vi "C-V measurement.vi"(5 "Session properties":T2, 7 "Workspace":path, 8 "Error In":errorcluster, 9 "myDLTS file path":path=path "", 10 "CV measurement":T22 {"CV properties"."Equivalent circuit model" items=["Rp || Cp", "Rs + Cs", "Rs + Ls", "G B", "D Cs", "Q Cs", "D Ls", "Q Ls", "Rp || Lp", "D Cp"]; "CV properties"."V range" items=["10mV"=0.01, "100mV"=0.1, "1V"=1.0, "10V"=10.0]; "CV properties"."I range" items=["100nA"=-7.0, "1µA"=-6.0, "10µA"=-5.0, "100µA"=-4.0, "1mA"=-3.0, "10mA"=-2.0]}, 11 "Loop data":T3={"Persistent"={"Last file"=path "", "Last user"="", "Users"=[]}, "Temp handle"={"Connected"=FALSE, "Temp ctrl"={"Gain (P)"=0.0, "Reset (I)"=0.0, "Rate (D)"=0.0, "Stabilization rate"=0.0, "Stabilization delta"=0.0, "Type"=enum."Lake Shore 325", "Custom temp ctrl"={"VISA resource name"=""}, "Lakeshore 325"={"VISA name"="", "Loop"=0, "Heater Range"=1, "Heater Resistance"=0, "Sample sensor"=0, "Fast sensor"=0, "Slow sensor"=0}, "Lakeshore 331"={"VISA name"="", "Loop"=1, "Heater Range"=0, "Sample sensor"=0, "Fast sensor"=0, "Slow sensor"=0}, "Lakeshore 332"={"VISA name"="", "Loop"=1, "Heater Range"=0, "Sample sensor"=0, "Fast sensor"=0, "Slow sensor"=0}, "Lakeshore 335"={"VISA name"="", "Loop"=1, "Sample sensor"=0, "Fast sensor"=0, "Slow sensor"=0, "Heater Range"=0, "Output mode"=enum."Off"}, "Lakeshore 336"={"VISA name"="", "Loop"=1, "Output mode"=enum."Off", "Max current"=1.0, "Heater resistance"=1, "Sample sensor"=1, "Slow sensor"=1, "Fast sensor"=1}}}, "Paths"={"Manual"=path "", "Settings"=path "", "Persistent"=path "", "Work dir."=path ""}, "Settings"={"MFIA"={"Address"="", "Use compensation"=TRUE, "Shut down gracefully"=FALSE}, "Temp ctrl"={"Gain (P)"=0.0, "Reset (I)"=0.0, "Rate (D)"=0.0, "Stabilization rate"=0.0, "Stabilization delta"=0.0, "Type"=enum."Lake Shore 325", "Custom temp ctrl"={"VISA resource name"=""}, "Lakeshore 325"={"VISA name"="", "Loop"=0, "Heater Range"=1, "Heater Resistance"=0, "Sample sensor"=0, "Fast sensor"=0, "Slow sensor"=0}, "Lakeshore 331"={"VISA name"="", "Loop"=1, "Heater Range"=0, "Sample sensor"=0, "Fast sensor"=0, "Slow sensor"=0}, "Lakeshore 332"={"VISA name"="", "Loop"=1, "Heater Range"=0, "Sample sensor"=0, "Fast sensor"=0, "Slow sensor"=0}, "Lakeshore 335"={"VISA name"="", "Loop"=1, "Sample sensor"=0, "Fast sensor"=0, "Slow sensor"=0, "Heater Range"=0, "Output mode"=enum."Off"}, "Lakeshore 336"={"VISA name"="", "Loop"=1, "Output mode"=enum."Off", "Max current"=1.0, "Heater resistance"=1, "Sample sensor"=1, "Slow sensor"=1, "Fast sensor"=1}}, "Source-meter"={"Type"=enum."Custom", "Custom source-meter"={"VISA resource name"=""}, "Keithley 2600"={"VISA name"="", "Ignore ID Query"=FALSE, "SMU"=enum."Channel A"}, "Keithley 2400 Series"={"VISA name"="", "Ignore ID Query"=FALSE}}, "Other"={"Enable OriginLab"=FALSE, "Reader mode"=FALSE, "Auto-save"=FALSE}, "Defaults"={"IV properties"={"T"=0.0, "Vstart"=-0.5, "Vstop"=0.5, "Vpoints"=10.0, "Settling"=0.01, "I limit"=0.1, "Log mapping"=FALSE, "Averaging"=0.0}, "CV properties"={"T"=0.0, "Vstart"=-0.5, "Vstop"=0.5, "Vpoints"=10.0, "Precision"=enum."Normal", "Test signal"=0.01, "Auto I range"=FALSE, "Test frequency"=100000.0, "I range"=-2.0, "V range"=10.0, "Log mapping"=FALSE, "Rel perm"=0.0, "Area"=0.0, "Equivalent circuit model"=0}, "DLTS properties"={"Tstart"=0.0, "Instant start"=FALSE, "Tstop"=0.0, "T rate"=0.0, "Test signal"=0.0, "Test frequency"=0.0, "Bandwidth"=0.0, "Averaging"=0.0, "Vbias"=0.0, "Vpulse"=0.0, "pulse length"=0.0, "Pulse 2"=FALSE, "Vpulse 2"=0.0, "pulse length 2"=0.0, "I range"=-2.0, "V range"=10.0, "Emission rate"=[], "Sampling rate"=0.0, "Acq. delay"=0.0, "Filter order"=0, "Equivalent circuit model"=0}, "LDLTS properties"={"T"=0.0, "Test signal"=0.0, "Test frequency"=0.0, "Bandwidth"=0.0, "Averaging"=0.0, "Vbias"=0.0, "Vpulse"=0.0, "pulse length"=0.0, "Pulse 2"=FALSE, "Vpulse 2"=0.0, "pulse length 2"=0.0, "I range"=-2.0, "V range"=10.0, "Sampling rate"=0.0, "Acq. delay"=0.0, "Sampling time"=0.0, "Filter order"=0, "Equivalent circuit model"=0}}}, "Software version"=0.0, "MFIA handle"={"ziHandle"={"handleValid"=FALSE, "Conn"=0, "Path Prefix"="", "Handle"=0, "Connected"=FALSE, "Clockbase(s)"=0.0}, "Selected device"="", "ziModHandle"={"handleValid"=FALSE, "Conn"=0, "ModHandle"=0, "moduleID"="", "Path Prefix"=""}}, "Source-meter handle"={"Connected"=FALSE, "Source-meter"={"Type"=enum."Custom", "Custom source-meter"={"VISA resource name"=""}, "Keithley 2600"={"VISA name"="", "Ignore ID Query"=FALSE, "SMU"=enum."Channel A"}, "Keithley 2400 Series"={"VISA name"="", "Ignore ID Query"=FALSE}}}} {"MFIA handle"."ziModHandle"."ModHandle" format="0x%08x"; "MFIA handle"."ziModHandle"."Conn" format="0x%08x"; "MFIA handle"."ziHandle"."Handle" format="0x%08x"; "MFIA handle"."ziHandle"."Conn" format="0x%08x"; "Settings"."Defaults"."LDLTS properties"."Equivalent circuit model" items=["Rp || Cp", "Rs + Cs", "Rs + Ls", "G B", "D Cs", "Q Cs", "D Ls", "Q Ls", "Rp || Lp", "D Cp"]; "Settings"."Defaults"."LDLTS properties"."Filter order" min=0 max=8 step=1; "Settings"."Defaults"."LDLTS properties"."Sampling rate" items=["13k"=13392.857422, "27k"=26785.714844, "54k"=53571.429687, "107k"=107142.859375]; "Settings"."Defaults"."LDLTS properties"."V range" items=["10mV"=0.01, "100mV"=0.1, "1V"=1.0, "10V"=10.0]; "Settings"."Defaults"."LDLTS properties"."I range" items=["100nA"=-7.0, "1µA"=-6.0, "10µA"=-5.0, "100µA"=-4.0, "1mA"=-3.0, "10mA"=-2.0]; "Settings"."Defaults"."DLTS properties"."Equivalent circuit model" items=["Rp || Cp", "Rs + Cs", "Rs + Ls", "G B", "D Cs", "Q Cs", "D Ls", "Q Ls", "Rp || Lp", "D Cp"]; "Settings"."Defaults"."DLTS properties"."Filter order" min=0 max=8 step=1; "Settings"."Defaults"."DLTS properties"."Sampling rate" items=["13k"=13392.857422, "27k"=26785.714844, "54k"=53571.429687, "107k"=107142.859375]; "Settings"."Defaults"."DLTS properties"."V range" items=["10mV"=0.01, "100mV"=0.1, "1V"=1.0, "10V"=10.0]; "Settings"."Defaults"."DLTS properties"."I range" items=["10mV"=0.01, "100mV"=0.1, "1V"=1.0, "10V"=10.0]; "Settings"."Defaults"."CV properties"."Equivalent circuit model" items=["Rp || Cp", "Rs + Cs", "Rs + Ls", "G B", "D Cs", "Q Cs", "D Ls", "Q Ls", "Rp || Lp", "D Cp"]; "Settings"."Defaults"."CV properties"."V range" items=["10mV"=0.01, "100mV"=0.1, "1V"=1.0, "10V"=10.0]; "Settings"."Defaults"."CV properties"."I range" items=["100nA"=-7.0, "1µA"=-6.0, "10µA"=-5.0, "100µA"=-4.0, "1mA"=-3.0, "10mA"=-2.0]; "Settings"."Defaults"."IV properties"."Settling" min=0.0 max=65535.0; "Settings"."Temp ctrl"."Lakeshore 336"."Fast sensor" items=["Sensor A", "Sensor B", "Sensor C", "Sensor D"]; "Settings"."Temp ctrl"."Lakeshore 336"."Slow sensor" items=["Sensor A", "Sensor B", "Sensor C", "Sensor D"]; "Settings"."Temp ctrl"."Lakeshore 336"."Sample sensor" items=["Sensor A", "Sensor B", "Sensor C", "Sensor D"]; "Settings"."Temp ctrl"."Lakeshore 336"."Heater resistance" items=["25 Ohm"=1, "50 Ohm"=2]; "Settings"."Temp ctrl"."Lakeshore 336"."Max current" items=["0.707 A"=0.0, "1 A"=1.0, "1.414 A"=1.414, "2 A"=2.0]; "Settings"."Temp ctrl"."Lakeshore 336"."Loop" items=["Output 1"=1, "Output 2"=2, "Output 3"=3, "Output 4"=4]; "Settings"."Temp ctrl"."Lakeshore 335"."Heater Range" items=["Off", "Low (On)", "Medium", "High"]; "Settings"."Temp ctrl"."Lakeshore 335"."Slow sensor" items=["A", "B"]; "Settings"."Temp ctrl"."Lakeshore 335"."Fast sensor" items=["A", "B"]; "Settings"."Temp ctrl"."Lakeshore 335"."Sample sensor" items=["A", "B"]; "Settings"."Temp ctrl"."Lakeshore 335"."Loop" items=["Loop 1"=1, "Loop 2"=2]; "Settings"."Temp ctrl"."Lakeshore 332"."Slow sensor" items=["A", "B"]; "Settings"."Temp ctrl"."Lakeshore 332"."Fast sensor" items=["A", "B"]; "Settings"."Temp ctrl"."Lakeshore 332"."Sample sensor" items=["A", "B"]; "Settings"."Temp ctrl"."Lakeshore 332"."Heater Range" items=["Off", "Low (0.5W)", "Med (5W)", "High (50W)"]; "Settings"."Temp ctrl"."Lakeshore 332"."Loop" items=["Loop 1", "Loop 2"]; "Settings"."Temp ctrl"."Lakeshore 331"."Slow sensor" items=["A", "B"]; "Settings"."Temp ctrl"."Lakeshore 331"."Fast sensor" items=["A", "B"]; "Settings"."Temp ctrl"."Lakeshore 331"."Sample sensor" items=["A", "B"]; "Settings"."Temp ctrl"."Lakeshore 331"."Heater Range" items=["Off", "Low (0.5W)", "Med (5W)", "High (50W)"]; "Settings"."Temp ctrl"."Lakeshore 331"."Loop" items=["Loop 1", "Loop 2"]; "Settings"."Temp ctrl"."Lakeshore 325"."Slow sensor" items=["A", "B"]; "Settings"."Temp ctrl"."Lakeshore 325"."Fast sensor" items=["A", "B"]; "Settings"."Temp ctrl"."Lakeshore 325"."Sample sensor" items=["A", "B"]; "Settings"."Temp ctrl"."Lakeshore 325"."Heater Resistance" items=["25 Ohm"=1, "50 Ohm"=2]; "Settings"."Temp ctrl"."Lakeshore 325"."Heater Range" items=["Off", "Low (loop 1) or On (loop 2)", "High (loop 1)"]; "Settings"."Temp ctrl"."Lakeshore 325"."Loop" items=["Loop 1"=1, "Loop 2"=2]; "Temp handle"."Temp ctrl"."Lakeshore 336"."Fast sensor" items=["Sensor A", "Sensor B", "Sensor C", "Sensor D"]; "Temp handle"."Temp ctrl"."Lakeshore 336"."Slow sensor" items=["Sensor A", "Sensor B", "Sensor C", "Sensor D"]; "Temp handle"."Temp ctrl"."Lakeshore 336"."Sample sensor" items=["Sensor A", "Sensor B", "Sensor C", "Sensor D"]; "Temp handle"."Temp ctrl"."Lakeshore 336"."Heater resistance" items=["25 Ohm"=1, "50 Ohm"=2]; "Temp handle"."Temp ctrl"."Lakeshore 336"."Max current" items=["0.707 A"=0.0, "1 A"=1.0, "1.414 A"=1.414, "2 A"=2.0]; "Temp handle"."Temp ctrl"."Lakeshore 336"."Loop" items=["Output 1"=1, "Output 2"=2, "Output 3"=3, "Output 4"=4]; "Temp handle"."Temp ctrl"."Lakeshore 335"."Heater Range" items=["Off", "Low (On)", "Medium", "High"]; "Temp handle"."Temp ctrl"."Lakeshore 335"."Slow sensor" items=["A", "B"]; "Temp handle"."Temp ctrl"."Lakeshore 335"."Fast sensor" items=["A", "B"]; "Temp handle"."Temp ctrl"."Lakeshore 335"."Sample sensor" items=["A", "B"]; "Temp handle"."Temp ctrl"."Lakeshore 335"."Loop" items=["Loop 1"=1, "Loop 2"=2]; "Temp handle"."Temp ctrl"."Lakeshore 332"."Slow sensor" items=["A", "B"]; "Temp handle"."Temp ctrl"."Lakeshore 332"."Fast sensor" items=["A", "B"]; "Temp handle"."Temp ctrl"."Lakeshore 332"."Sample sensor" items=["A", "B"]; "Temp handle"."Temp ctrl"."Lakeshore 332"."Heater Range" items=["Off", "Low (0.5W)", "Med (5W)", "High (50W)"]; "Temp handle"."Temp ctrl"."Lakeshore 332"."Loop" items=["Loop 1", "Loop 2"]; "Temp handle"."Temp ctrl"."Lakeshore 331"."Slow sensor" items=["A", "B"]; "Temp handle"."Temp ctrl"."Lakeshore 331"."Fast sensor" items=["A", "B"]; "Temp handle"."Temp ctrl"."Lakeshore 331"."Sample sensor" items=["A", "B"]; "Temp handle"."Temp ctrl"."Lakeshore 331"."Heater Range" items=["Off", "Low (0.5W)", "Med (5W)", "High (50W)"]; "Temp handle"."Temp ctrl"."Lakeshore 331"."Loop" items=["Loop 1", "Loop 2"]; "Temp handle"."Temp ctrl"."Lakeshore 325"."Slow sensor" items=["A", "B"]; "Temp handle"."Temp ctrl"."Lakeshore 325"."Fast sensor" items=["A", "B"]; "Temp handle"."Temp ctrl"."Lakeshore 325"."Sample sensor" items=["A", "B"]; "Temp handle"."Temp ctrl"."Lakeshore 325"."Heater Resistance" items=["25 Ohm"=1, "50 Ohm"=2]; "Temp handle"."Temp ctrl"."Lakeshore 325"."Heater Range" items=["Off", "Low (loop 1) or On (loop 2)", "High (loop 1)"]; "Temp handle"."Temp ctrl"."Lakeshore 325"."Loop" items=["Loop 1"=1, "Loop 2"=2]}) -> (0 "Error Out":errorcluster, 1 "Modified":bool, 2 "CV measurement out":T22 {"CV properties"."Equivalent circuit model" items=["Rp || Cp", "Rs + Cs", "Rs + Ls", "G B", "D Cs", "Q Cs", "D Ls", "Q Ls", "Rp || Lp", "D Cp"]; "CV properties"."V range" items=["10mV"=0.01, "100mV"=0.1, "1V"=1.0, "10V"=10.0]; "CV properties"."I range" items=["100nA"=-7.0, "1µA"=-6.0, "10µA"=-5.0, "100µA"=-4.0, "1mA"=-3.0, "10mA"=-2.0]}, 3 "Loop data out":T3={"Persistent"={"Last file"=path "", "Last user"="", "Users"=[]}, "Temp handle"={"Connected"=FALSE, "Temp ctrl"={"Gain (P)"=0.0, "Reset (I)"=0.0, "Rate (D)"=0.0, "Stabilization rate"=0.0, "Stabilization delta"=0.0, "Type"=enum."Lake Shore 325", "Custom temp ctrl"={"VISA resource name"=""}, "Lakeshore 325"={"VISA name"="", "Loop"=0, "Heater Range"=1, "Heater Resistance"=0, "Sample sensor"=0, "Fast sensor"=0, "Slow sensor"=0}, "Lakeshore 331"={"VISA name"="", "Loop"=1, "Heater Range"=0, "Sample sensor"=0, "Fast sensor"=0, "Slow sensor"=0}, "Lakeshore 332"={"VISA name"="", "Loop"=1, "Heater Range"=0, "Sample sensor"=0, "Fast sensor"=0, "Slow sensor"=0}, "Lakeshore 335"={"VISA name"="", "Loop"=1, "Sample sensor"=0, "Fast sensor"=0, "Slow sensor"=0, "Heater Range"=0, "Output mode"=enum."Off"}, "Lakeshore 336"={"VISA name"="", "Loop"=1, "Output mode"=enum."Off", "Max current"=1.0, "Heater resistance"=1, "Sample sensor"=1, "Slow sensor"=1, "Fast sensor"=1}}}, "Paths"={"Manual"=path "", "Settings"=path "", "Persistent"=path "", "Work dir."=path ""}, "Settings"={"MFIA"={"Address"="", "Use compensation"=TRUE, "Shut down gracefully"=FALSE}, "Temp ctrl"={"Gain (P)"=0.0, "Reset (I)"=0.0, "Rate (D)"=0.0, "Stabilization rate"=0.0, "Stabilization delta"=0.0, "Type"=enum."Lake Shore 325", "Custom temp ctrl"={"VISA resource name"=""}, "Lakeshore 325"={"VISA name"="", "Loop"=0, "Heater Range"=1, "Heater Resistance"=0, "Sample sensor"=0, "Fast sensor"=0, "Slow sensor"=0}, "Lakeshore 331"={"VISA name"="", "Loop"=1, "Heater Range"=0, "Sample sensor"=0, "Fast sensor"=0, "Slow sensor"=0}, "Lakeshore 332"={"VISA name"="", "Loop"=1, "Heater Range"=0, "Sample sensor"=0, "Fast sensor"=0, "Slow sensor"=0}, "Lakeshore 335"={"VISA name"="", "Loop"=1, "Sample sensor"=0, "Fast sensor"=0, "Slow sensor"=0, "Heater Range"=0, "Output mode"=enum."Off"}, "Lakeshore 336"={"VISA name"="", "Loop"=1, "Output mode"=enum."Off", "Max current"=1.0, "Heater resistance"=1, "Sample sensor"=1, "Slow sensor"=1, "Fast sensor"=1}}, "Source-meter"={"Type"=enum."Custom", "Custom source-meter"={"VISA resource name"=""}, "Keithley 2600"={"VISA name"="", "Ignore ID Query"=FALSE, "SMU"=enum."Channel A"}, "Keithley 2400 Series"={"VISA name"="", "Ignore ID Query"=FALSE}}, "Other"={"Enable OriginLab"=FALSE, "Reader mode"=FALSE, "Auto-save"=FALSE}, "Defaults"={"IV properties"={"T"=0.0, "Vstart"=-0.5, "Vstop"=0.5, "Vpoints"=10.0, "Settling"=0.01, "I limit"=0.1, "Log mapping"=FALSE, "Averaging"=0.0}, "CV properties"={"T"=0.0, "Vstart"=-0.5, "Vstop"=0.5, "Vpoints"=10.0, "Precision"=enum."Normal", "Test signal"=0.01, "Auto I range"=FALSE, "Test frequency"=100000.0, "I range"=-2.0, "V range"=10.0, "Log mapping"=FALSE, "Rel perm"=0.0, "Area"=0.0, "Equivalent circuit model"=0}, "DLTS properties"={"Tstart"=0.0, "Instant start"=FALSE, "Tstop"=0.0, "T rate"=0.0, "Test signal"=0.0, "Test frequency"=0.0, "Bandwidth"=0.0, "Averaging"=0.0, "Vbias"=0.0, "Vpulse"=0.0, "pulse length"=0.0, "Pulse 2"=FALSE, "Vpulse 2"=0.0, "pulse length 2"=0.0, "I range"=-2.0, "V range"=10.0, "Emission rate"=[], "Sampling rate"=0.0, "Acq. delay"=0.0, "Filter order"=0, "Equivalent circuit model"=0}, "LDLTS properties"={"T"=0.0, "Test signal"=0.0, "Test frequency"=0.0, "Bandwidth"=0.0, "Averaging"=0.0, "Vbias"=0.0, "Vpulse"=0.0, "pulse length"=0.0, "Pulse 2"=FALSE, "Vpulse 2"=0.0, "pulse length 2"=0.0, "I range"=-2.0, "V range"=10.0, "Sampling rate"=0.0, "Acq. delay"=0.0, "Sampling time"=0.0, "Filter order"=0, "Equivalent circuit model"=0}}}, "Software version"=0.0, "MFIA handle"={"ziHandle"={"handleValid"=FALSE, "Conn"=0, "Path Prefix"="", "Handle"=0, "Connected"=FALSE, "Clockbase(s)"=0.0}, "Selected device"="", "ziModHandle"={"handleValid"=FALSE, "Conn"=0, "ModHandle"=0, "moduleID"="", "Path Prefix"=""}}, "Source-meter handle"={"Connected"=FALSE, "Source-meter"={"Type"=enum."Custom", "Custom source-meter"={"VISA resource name"=""}, "Keithley 2600"={"VISA name"="", "Ignore ID Query"=FALSE, "SMU"=enum."Channel A"}, "Keithley 2400 Series"={"VISA name"="", "Ignore ID Query"=FALSE}}}} {"MFIA handle"."ziModHandle"."ModHandle" format="0x%08x"; "MFIA handle"."ziModHandle"."Conn" format="0x%08x"; "MFIA handle"."ziHandle"."Handle" format="0x%08x"; "MFIA handle"."ziHandle"."Conn" format="0x%08x"; "Settings"."Defaults"."LDLTS properties"."Equivalent circuit model" items=["Rp || Cp", "Rs + Cs", "Rs + Ls", "G B", "D Cs", "Q Cs", "D Ls", "Q Ls", "Rp || Lp", "D Cp"]; "Settings"."Defaults"."LDLTS properties"."Filter order" min=0 max=8 step=1; "Settings"."Defaults"."LDLTS properties"."Sampling rate" items=["13k"=13392.857422, "27k"=26785.714844, "54k"=53571.429687, "107k"=107142.859375]; "Settings"."Defaults"."LDLTS properties"."V range" items=["10mV"=0.01, "100mV"=0.1, "1V"=1.0, "10V"=10.0]; "Settings"."Defaults"."LDLTS properties"."I range" items=["100nA"=-7.0, "1µA"=-6.0, "10µA"=-5.0, "100µA"=-4.0, "1mA"=-3.0, "10mA"=-2.0]; "Settings"."Defaults"."DLTS properties"."Equivalent circuit model" items=["Rp || Cp", "Rs + Cs", "Rs + Ls", "G B", "D Cs", "Q Cs", "D Ls", "Q Ls", "Rp || Lp", "D Cp"]; "Settings"."Defaults"."DLTS properties"."Filter order" min=0 max=8 step=1; "Settings"."Defaults"."DLTS properties"."Sampling rate" items=["13k"=13392.857422, "27k"=26785.714844, "54k"=53571.429687, "107k"=107142.859375]; "Settings"."Defaults"."DLTS properties"."V range" items=["10mV"=0.01, "100mV"=0.1, "1V"=1.0, "10V"=10.0]; "Settings"."Defaults"."DLTS properties"."I range" items=["10mV"=0.01, "100mV"=0.1, "1V"=1.0, "10V"=10.0]; "Settings"."Defaults"."CV properties"."Equivalent circuit model" items=["Rp || Cp", "Rs + Cs", "Rs + Ls", "G B", "D Cs", "Q Cs", "D Ls", "Q Ls", "Rp || Lp", "D Cp"]; "Settings"."Defaults"."CV properties"."V range" items=["10mV"=0.01, "100mV"=0.1, "1V"=1.0, "10V"=10.0]; "Settings"."Defaults"."CV properties"."I range" items=["100nA"=-7.0, "1µA"=-6.0, "10µA"=-5.0, "100µA"=-4.0, "1mA"=-3.0, "10mA"=-2.0]; "Settings"."Defaults"."IV properties"."Settling" min=0.0 max=65535.0; "Settings"."Temp ctrl"."Lakeshore 336"."Fast sensor" items=["Sensor A", "Sensor B", "Sensor C", "Sensor D"]; "Settings"."Temp ctrl"."Lakeshore 336"."Slow sensor" items=["Sensor A", "Sensor B", "Sensor C", "Sensor D"]; "Settings"."Temp ctrl"."Lakeshore 336"."Sample sensor" items=["Sensor A", "Sensor B", "Sensor C", "Sensor D"]; "Settings"."Temp ctrl"."Lakeshore 336"."Heater resistance" items=["25 Ohm"=1, "50 Ohm"=2]; "Settings"."Temp ctrl"."Lakeshore 336"."Max current" items=["0.707 A"=0.0, "1 A"=1.0, "1.414 A"=1.414, "2 A"=2.0]; "Settings"."Temp ctrl"."Lakeshore 336"."Loop" items=["Output 1"=1, "Output 2"=2, "Output 3"=3, "Output 4"=4]; "Settings"."Temp ctrl"."Lakeshore 335"."Heater Range" items=["Off", "Low (On)", "Medium", "High"]; "Settings"."Temp ctrl"."Lakeshore 335"."Slow sensor" items=["A", "B"]; "Settings"."Temp ctrl"."Lakeshore 335"."Fast sensor" items=["A", "B"]; "Settings"."Temp ctrl"."Lakeshore 335"."Sample sensor" items=["A", "B"]; "Settings"."Temp ctrl"."Lakeshore 335"."Loop" items=["Loop 1"=1, "Loop 2"=2]; "Settings"."Temp ctrl"."Lakeshore 332"."Slow sensor" items=["A", "B"]; "Settings"."Temp ctrl"."Lakeshore 332"."Fast sensor" items=["A", "B"]; "Settings"."Temp ctrl"."Lakeshore 332"."Sample sensor" items=["A", "B"]; "Settings"."Temp ctrl"."Lakeshore 332"."Heater Range" items=["Off", "Low (0.5W)", "Med (5W)", "High (50W)"]; "Settings"."Temp ctrl"."Lakeshore 332"."Loop" items=["Loop 1", "Loop 2"]; "Settings"."Temp ctrl"."Lakeshore 331"."Slow sensor" items=["A", "B"]; "Settings"."Temp ctrl"."Lakeshore 331"."Fast sensor" items=["A", "B"]; "Settings"."Temp ctrl"."Lakeshore 331"."Sample sensor" items=["A", "B"]; "Settings"."Temp ctrl"."Lakeshore 331"."Heater Range" items=["Off", "Low (0.5W)", "Med (5W)", "High (50W)"]; "Settings"."Temp ctrl"."Lakeshore 331"."Loop" items=["Loop 1", "Loop 2"]; "Settings"."Temp ctrl"."Lakeshore 325"."Slow sensor" items=["A", "B"]; "Settings"."Temp ctrl"."Lakeshore 325"."Fast sensor" items=["A", "B"]; "Settings"."Temp ctrl"."Lakeshore 325"."Sample sensor" items=["A", "B"]; "Settings"."Temp ctrl"."Lakeshore 325"."Heater Resistance" items=["25 Ohm"=1, "50 Ohm"=2]; "Settings"."Temp ctrl"."Lakeshore 325"."Heater Range" items=["Off", "Low (loop 1) or On (loop 2)", "High (loop 1)"]; "Settings"."Temp ctrl"."Lakeshore 325"."Loop" items=["Loop 1"=1, "Loop 2"=2]; "Temp handle"."Temp ctrl"."Lakeshore 336"."Fast sensor" items=["Sensor A", "Sensor B", "Sensor C", "Sensor D"]; "Temp handle"."Temp ctrl"."Lakeshore 336"."Slow sensor" items=["Sensor A", "Sensor B", "Sensor C", "Sensor D"]; "Temp handle"."Temp ctrl"."Lakeshore 336"."Sample sensor" items=["Sensor A", "Sensor B", "Sensor C", "Sensor D"]; "Temp handle"."Temp ctrl"."Lakeshore 336"."Heater resistance" items=["25 Ohm"=1, "50 Ohm"=2]; "Temp handle"."Temp ctrl"."Lakeshore 336"."Max current" items=["0.707 A"=0.0, "1 A"=1.0, "1.414 A"=1.414, "2 A"=2.0]; "Temp handle"."Temp ctrl"."Lakeshore 336"."Loop" items=["Output 1"=1, "Output 2"=2, "Output 3"=3, "Output 4"=4]; "Temp handle"."Temp ctrl"."Lakeshore 335"."Heater Range" items=["Off", "Low (On)", "Medium", "High"]; "Temp handle"."Temp ctrl"."Lakeshore 335"."Slow sensor" items=["A", "B"]; "Temp handle"."Temp ctrl"."Lakeshore 335"."Fast sensor" items=["A", "B"]; "Temp handle"."Temp ctrl"."Lakeshore 335"."Sample sensor" items=["A", "B"]; "Temp handle"."Temp ctrl"."Lakeshore 335"."Loop" items=["Loop 1"=1, "Loop 2"=2]; "Temp handle"."Temp ctrl"."Lakeshore 332"."Slow sensor" items=["A", "B"]; "Temp handle"."Temp ctrl"."Lakeshore 332"."Fast sensor" items=["A", "B"]; "Temp handle"."Temp ctrl"."Lakeshore 332"."Sample sensor" items=["A", "B"]; "Temp handle"."Temp ctrl"."Lakeshore 332"."Heater Range" items=["Off", "Low (0.5W)", "Med (5W)", "High (50W)"]; "Temp handle"."Temp ctrl"."Lakeshore 332"."Loop" items=["Loop 1", "Loop 2"]; "Temp handle"."Temp ctrl"."Lakeshore 331"."Slow sensor" items=["A", "B"]; "Temp handle"."Temp ctrl"."Lakeshore 331"."Fast sensor" items=["A", "B"]; "Temp handle"."Temp ctrl"."Lakeshore 331"."Sample sensor" items=["A", "B"]; "Temp handle"."Temp ctrl"."Lakeshore 331"."Heater Range" items=["Off", "Low (0.5W)", "Med (5W)", "High (50W)"]; "Temp handle"."Temp ctrl"."Lakeshore 331"."Loop" items=["Loop 1", "Loop 2"]; "Temp handle"."Temp ctrl"."Lakeshore 325"."Slow sensor" items=["A", "B"]; "Temp handle"."Temp ctrl"."Lakeshore 325"."Fast sensor" items=["A", "B"]; "Temp handle"."Temp ctrl"."Lakeshore 325"."Sample sensor" items=["A", "B"]; "Temp handle"."Temp ctrl"."Lakeshore 325"."Heater Resistance" items=["25 Ohm"=1, "50 Ohm"=2]; "Temp handle"."Temp ctrl"."Lakeshore 325"."Heater Range" items=["Off", "Low (loop 1) or On (loop 2)", "High (loop 1)"]; "Temp handle"."Temp ctrl"."Lakeshore 325"."Loop" items=["Loop 1"=1, "Loop 2"=2]})   [LabVIEW 2019]
doc: "Handles C-V measurements, displays C-V masurement GUI window"
uses:
  Type defs/Loop data Type Def.ctl
  Type defs/Persistent Type Def.ctl
  Type defs/Temp handle Type Def.ctl
  Type defs/Temp ctrl Type Def.ctl
  Custom devices/Custom temp ctrl settings.ctl
  Type defs/Paths Type Def.ctl
  Type defs/Settings Type Def.ctl
  Type defs/Imps Type Def.ctl
  Type defs/Source-meter Type Def.ctl
  Custom devices/Custom source-meter settings.ctl
  Type defs/Other settings Type Def.ctl
  Type defs/IV properties Type Def.ctl
  Type defs/CV properties Type Def.ctl
  Type defs/DLTS properties Type Def.ctl
  Type defs/LDLTS properties Type Def.ctl
  Type defs/MFIA handle Type Def.ctl
  <instrlib>/Zurich Instruments LabOne/Public/ziTypeHandle.ctl
  <instrlib>/Zurich Instruments LabOne/Public/Modules/ziTypeModHandle.ctl
  Type defs/Source-meter handle Type Def.ctl
  Type defs/CV measurement Type Def.ctl
  Type defs/Session properties Type Def.ctl
  <vilib>/Utility/error.llb/DialogType.ctl
  <instrlib>/Zurich Instruments LabOne/Public/Modules/ziTypeModEnum.ctl
  <vilib>/event_ctls.llb/eventsource.ctl
  <instrlib>/Zurich Instruments LabOne/Public/Configure/ziSetValueDouble.vi
  <instrlib>/Zurich Instruments LabOne/Public/Modules/ziModSetValueBinaryArray.vi
  <instrlib>/Zurich Instruments LabOne/Public/Modules/ziModSetValueDoubleArray.vi
  <instrlib>/Zurich Instruments LabOne/Public/Modules/ziModGetSweeperData.vi
  Export single dat - CV cluster.vi
  Export single clipboard - CV cluster.vi
  Export Origin - CV.vi
  <instrlib>/Zurich Instruments LabOne/Zurich Instruments LabOne.lvlib
  <vilib>/Analysis/NI_AALPro.lvlib
panel:
  in  "Model":u16(ring) caption="Equivalent circuit model" items=["Rp || Cp", "Rs + Cs"]
  in  "Stop":bool
  in  "Folder":path
  in  "Calculate":bool
  in  "Rel perm":dbl=500.0 caption="Relative premittivity" min=0.0
  in  "Area":dbl[unit]=0.0005 caption="Junction area" min=0.0
  in  "Buttons":T1
  in  "Log mapping":bool caption="Log dist."
  out "Measurement info":string
  in  "V range":dbl[unit](ring)=10.0 caption="Voltage range" items=["10mV"=0.01, "100mV"=0.1, "1V"=1.0, "10V"=10.0]
  in  "Test frequency":dbl[unit]=100000.0 caption="Numeric" format="%#_6p"
  in  "I range":dbl(ring)=-7.0 caption="Current range" items=["100nA"=-7.0, "1µA"=-6.0, "10µA"=-5.0, "100µA"=-4.0, "1mA"=-3.0, "10mA"=-2.0]
  in  "Measure":bool
  in  "Voltage points":dbl=100.0 caption="Numeric"
  in  "End voltage":dbl[unit]=0.5 caption="Numeric" format="%#_6p"
  in  "Start voltage":dbl[unit]=-0.5 caption="Numeric" format="%#_6p"
  in  "Test signal":dbl[unit]=0.3 caption="Numeric" format="%#_6p"
  in  "Auto I range":bool=TRUE caption="Auto"
  in  "Precision":enum16{"Low (Fast)", "Normal", "High (Slow)"}(ring)=enum."Normal" caption="Enum"
  in  "Setpoint":dbl[unit]=1.0 caption="Numeric" min=1.0 max=800.0
  out "Temperature":dbl[unit] caption="Numeric"
  in  "Connect":bool
  out "C-V":cluster{"2D data":dbl[], "2D data":dbl[]}(graph)
  out "Concentration":cluster{sgl[], sgl[]}(graph)
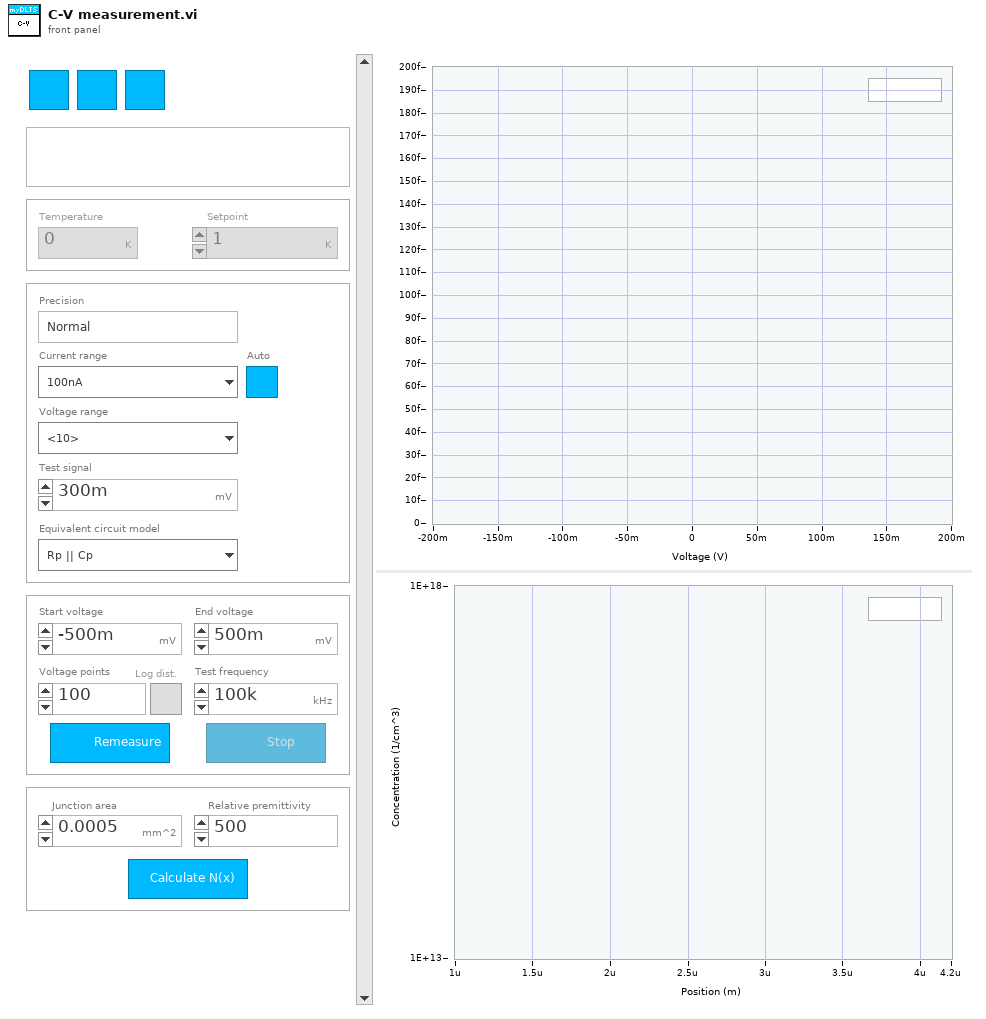
[diagram p1: front panel]
types:
  T1 = cluster{"Information":bool, "Help":bool, "Export":bool}
  T2 = typedef "Session properties Type Def.ctl" = cluster{"Session name":string, "Comment":string, "User":string, "Software version":dbl, "Created":timestamp, "Modified":timestamp, "Binary":bool, "GUID":string}
  T3 = typedef "Loop data Type Def.ctl" = cluster{"Persistent":T4, "Temp handle":T5, "Paths":T8, "Settings":T9, "Software version":dbl, "MFIA handle":T18, "Source-meter handle":T21}
  T4 = typedef "Persistent Type Def.ctl" = cluster{"Last file":path, "Last user":string, "Users":cluster{"User":string, "Authors directory":path}[]}
  T5 = typedef "Temp handle Type Def.ctl" = cluster{"Connected":bool, "Temp ctrl":T6}
  T6 = typedef "Temp ctrl Type Def.ctl" = cluster{"Gain (P)":dbl, "Reset (I)":dbl, "Rate (D)":dbl, "Stabilization rate":dbl, "Stabilization delta":dbl, "Type":enum16{"Custom", "Lake Shore 325", "Lake Shore 331", "Lake Shore 332", "Lake Shore 335", "Lake Shore 336"}, "Custom temp ctrl":T7, "Lakeshore 325":cluster{"VISA name":refnum<visa-resource-name>, "Loop":u16, "Heater Range":u16, "Heater Resistance":u16, "Sample sensor":u16, "Fast sensor":u16, "Slow sensor":u16}, "Lakeshore 331":cluster{"VISA name":refnum<visa-resource-name>, "Loop":u16, "Heater Range":u16, "Sample sensor":u16, "Fast sensor":u16, "Slow sensor":u16}, "Lakeshore 332":cluster{"VISA name":refnum<visa-resource-name>, "Loop":u16, "Heater Range":u16, "Sample sensor":u16, "Fast sensor":u16, "Slow sensor":u16}, "Lakeshore 335":cluster{"VISA name":refnum<visa-resource-name>, "Loop":u16, "Sample sensor":u16, "Fast sensor":u16, "Slow sensor":u16, "Heater Range":u16, "Output mode":enum16{"Off", "Closed Loop PID", "Zone", "Open Loop", "Monitor Out", "Warmup Supply"}}, "Lakeshore 336":cluster{"VISA name":refnum<visa-resource-name>, "Loop":u16, "Output mode":enum16{"Off", "Closed Loop PID", "Zone", "Open Loop"}, "Max current":dbl, "Heater resistance":u16, "Sample sensor":u16, "Slow sensor":u16, "Fast sensor":u16}}
  T7 = typedef "Custom temp ctrl settings.ctl" = cluster{"VISA resource name":refnum<visa-resource-name>}
  T8 = typedef "Paths Type Def.ctl" = cluster{"Manual":path, "Settings":path, "Persistent":path, "Work dir.":path}
  T9 = typedef "Settings Type Def.ctl" = cluster{"MFIA":T10, "Temp ctrl":T6, "Source-meter":T11, "Other":T13, "Defaults":cluster{"IV properties":T14, "CV properties":T15, "DLTS properties":T16, "LDLTS properties":T17}}
  T10 = typedef "Imps Type Def.ctl" = cluster{"Address":string, "Use compensation":bool, "Shut down gracefully":bool}
  T11 = typedef "Source-meter Type Def.ctl" = cluster{"Type":enum16{"Custom", "Keithley 2600", "Keithley 2400 Series"}, "Custom source-meter":T12, "Keithley 2600":cluster{"VISA name":refnum<visa-resource-name>, "Ignore ID Query":bool, "SMU":enum16{"Channel A", "Channel B"}}, "Keithley 2400 Series":cluster{"VISA name":refnum<visa-resource-name>, "Ignore ID Query":bool}}
  T12 = typedef "Custom source-meter settings.ctl" = cluster{"VISA resource name":refnum<visa-resource-name>}
  T13 = typedef "Other settings Type Def.ctl" = cluster{"Enable OriginLab":bool, "Reader mode":bool, "Auto-save":bool}
  T14 = typedef "IV properties Type Def.ctl" = cluster{"T":dbl[unit], "Vstart":dbl[unit], "Vstop":dbl[unit], "Vpoints":dbl, "Settling":dbl[unit], "I limit":dbl[unit], "Log mapping":bool, "Averaging":dbl}
  T15 = typedef "CV properties Type Def.ctl" = cluster{"T":dbl[unit], "Vstart":dbl[unit], "Vstop":dbl[unit], "Vpoints":dbl, "Precision":enum16{"Low (Fast)", "Normal", "High (Slow)"}, "Test signal":dbl[unit], "Auto I range":bool, "Test frequency":dbl[unit], "I range":dbl, "V range":dbl[unit], "Log mapping":bool, "Rel perm":dbl, "Area":dbl[unit], "Equivalent circuit model":u16}
  T16 = typedef "DLTS properties Type Def.ctl" = cluster{"Tstart":dbl[unit], "Instant start":bool, "Tstop":dbl[unit], "T rate":dbl[unit], "Test signal":dbl[unit], "Test frequency":dbl[unit], "Bandwidth":dbl[unit], "Averaging":dbl, "Vbias":dbl[unit], "Vpulse":dbl[unit], "pulse length":dbl[unit], "Pulse 2":bool, "Vpulse 2":dbl[unit], "pulse length 2":dbl[unit], "I range":dbl, "V range":dbl[unit], "Emission rate":dbl[unit][], "Sampling rate":dbl[unit], "Acq. delay":dbl[unit], "Filter order":i32, "Equivalent circuit model":u16}
  T17 = typedef "LDLTS properties Type Def.ctl" = cluster{"T":dbl[unit], "Test signal":dbl[unit], "Test frequency":dbl[unit], "Bandwidth":dbl[unit], "Averaging":dbl, "Vbias":dbl[unit], "Vpulse":dbl[unit], "pulse length":dbl[unit], "Pulse 2":bool, "Vpulse 2":dbl[unit], "pulse length 2":dbl[unit], "I range":dbl, "V range":dbl[unit], "Sampling rate":dbl[unit], "Acq. delay":dbl[unit], "Sampling time":dbl[unit], "Filter order":i32, "Equivalent circuit model":u16}
  T18 = typedef "MFIA handle Type Def.ctl" = cluster{"ziHandle":T19, "Selected device":string, "ziModHandle":T20}
  T19 = typedef "Zurich Instruments LabOne.lvlib/ziTypeHandle.ctl" = cluster{"handleValid":bool, "Conn":u64, "Path Prefix":string, "Handle":u64, "Connected":bool, "Clockbase(s)":dbl}
  T20 = typedef "Zurich Instruments LabOne.lvlib/ziTypeModHandle.ctl" = cluster{"handleValid":bool, "Conn":u64, "ModHandle":u64, "moduleID":string, "Path Prefix":string}
  T21 = typedef "Source-meter handle Type Def.ctl" = cluster{"Connected":bool, "Source-meter":T11}
  T22 = typedef "CV measurement Type Def.ctl" = cluster{"Name":string, "Comment":string, "Time":timestamp, "Folder":path, "CV properties":T15, "GUID":string}
  T23 = cluster{"MFIA":bool, "Temperature controller":bool, "Source meter":bool}
  T24 = enum8{"Enabled", "Disabled", "Disabled and Grayed Out"}
  T25 = cluster{"Clipboard":bool, "dat":bool, "iso":bool, "Origin":bool, "Excel":bool}
  T26 = typedef "DialogType.ctl" = u16
  T27 = typedef "eventsource.ctl" = u32
  T28 = enum16{"Canceled", "Clipboard", "Dat", "Iso", "Origin", "Excel"}
  T29 = cluster{"model":u16, "auto/output":bool, "output/amplitude":dbl, "current/range":dbl, "voltage/range":dbl, "auto/inputrange":bool, "mode":u16}
  T30 = typedef "Zurich Instruments LabOne.lvlib/ziTypeModEnum.ctl" = u16
  T31 = typedef "Zurich Instruments LabOne.lvlib/ziTypeModResults.ctl" = cluster{"PathArray":string[], "ValueType":T32, "NoOfResults":u64, "ziGenericHeader":T33[]}
  T32 = typedef "Zurich Instruments LabOne.lvlib/ziTypePollType.ctl" = enum16{"NONE", "DOUBLE_DATA", "INTEGER_DATA", "DEMOD_SAMPLE", "SCOPE_WAVE_HF2", "AUXIN_SAMPLE", "DIO_SAMPLE", "BYTE_ARRAY", "PWA_WAVE", "9", "10", "11", "12", "13", "14", "15", "TREE_CHANGE_DEPRI", "17", "ERROR", "19", "20", "21", "22", "23", "24", "25", "26", "27", "28", "29", "30", "31", "DOUBLE_DATA_TS", "INTEGER_DATA_TS", "34", "SCOPE_WAVE", "SCOPE_WAVE_EX", "37", "BYTE_ARRAY_TS", "39", "40", "41", "42", "43", "44", "45", "CNT_DATA", "47", "TREE_CHANGE", "49", "50", "51", "52", "53", "54", "55", "56", "57", "58", "59", "60", "61", "62", "63", "SWEEPER_DATA", "SPECTRUM_DATA", "ADVISOR_DATA", "VECTOR_DATA", "IMP_DATA", "SHF_GENERATOR_WAVEFORM_DATA", "SHF_RESULT_LOGGER_DATA", "SHF_SCOPE_DATA", "DEMOD_VECTOR"}
  T33 = typedef "Zurich Instruments LabOne.lvlib/ziTypeModGenericHeader.ctl" = cluster{"HeaderType":enum8{"HEADER_TYPE_NONE", "HEADER_TYPE_SWTRIGGER", "HEADER_TYPE_SWEEPER"}, "SampleFormat":u8, "SystemTime":timestamp, "CreatedTimeStamp":u64, "ChangedTimeStamp":u64, "Flags":u32, "ChunkSizeBytes":u64, "Name":string, "Status":u32, "GroupIndex":u32, "Color":u32, "ActiveRow":u32, "TriggerNumber":u64, "GridRows":u32, "GridCols":u32, "GridMode":u32, "GridOperation":u32, "GridDirection":u32, "GridRepetitions":u32, "GridColDelta":dbl, "GridColOffset":dbl, "GridRowDelta":dbl, "GridRowOffset":dbl, "Bandwidth":dbl, "Center":dbl, "Nenbw":dbl}
  T34 = typedef "Zurich Instruments LabOne.lvlib/ziTypeModSweeperImpedanceWave.ctl" = cluster{"timestamp":u64, "sampleCount":u64, "flags":u8, "sampleFormat":u8, "sweepMode":u8, "bandwidthMode":u8, "count":u64[], "settimestamp":u64[], "nexttimestamp":u64[], "grid":dbl[], "bandwidth":dbl[], "tc":dbl[], "tcmeas":dbl[], "settling":dbl[], "realz":dbl[], "realzstddev":dbl[], "realzpwr":dbl[], "imagz":dbl[], "imagzstddev":dbl[], "imagzpwr":dbl[], "absz":dbl[], "abszstddev":dbl[], "abszpwr":dbl[], "phasez":dbl[], "phasezstddev":dbl[], "phasezpwr":dbl[], "frequency":dbl[], "frequencystddev":dbl[], "frequencypwr":dbl[], "param0":dbl[], "param0stddev":dbl[], "param0pwr":dbl[], "param1":dbl[], "param1stddev":dbl[], "param1pwr":dbl[], "drive":dbl[], "drivestddev":dbl[], "drivepwr":dbl[], "bias":dbl[], "biasstddev":dbl[], "biaspwr":dbl[]}
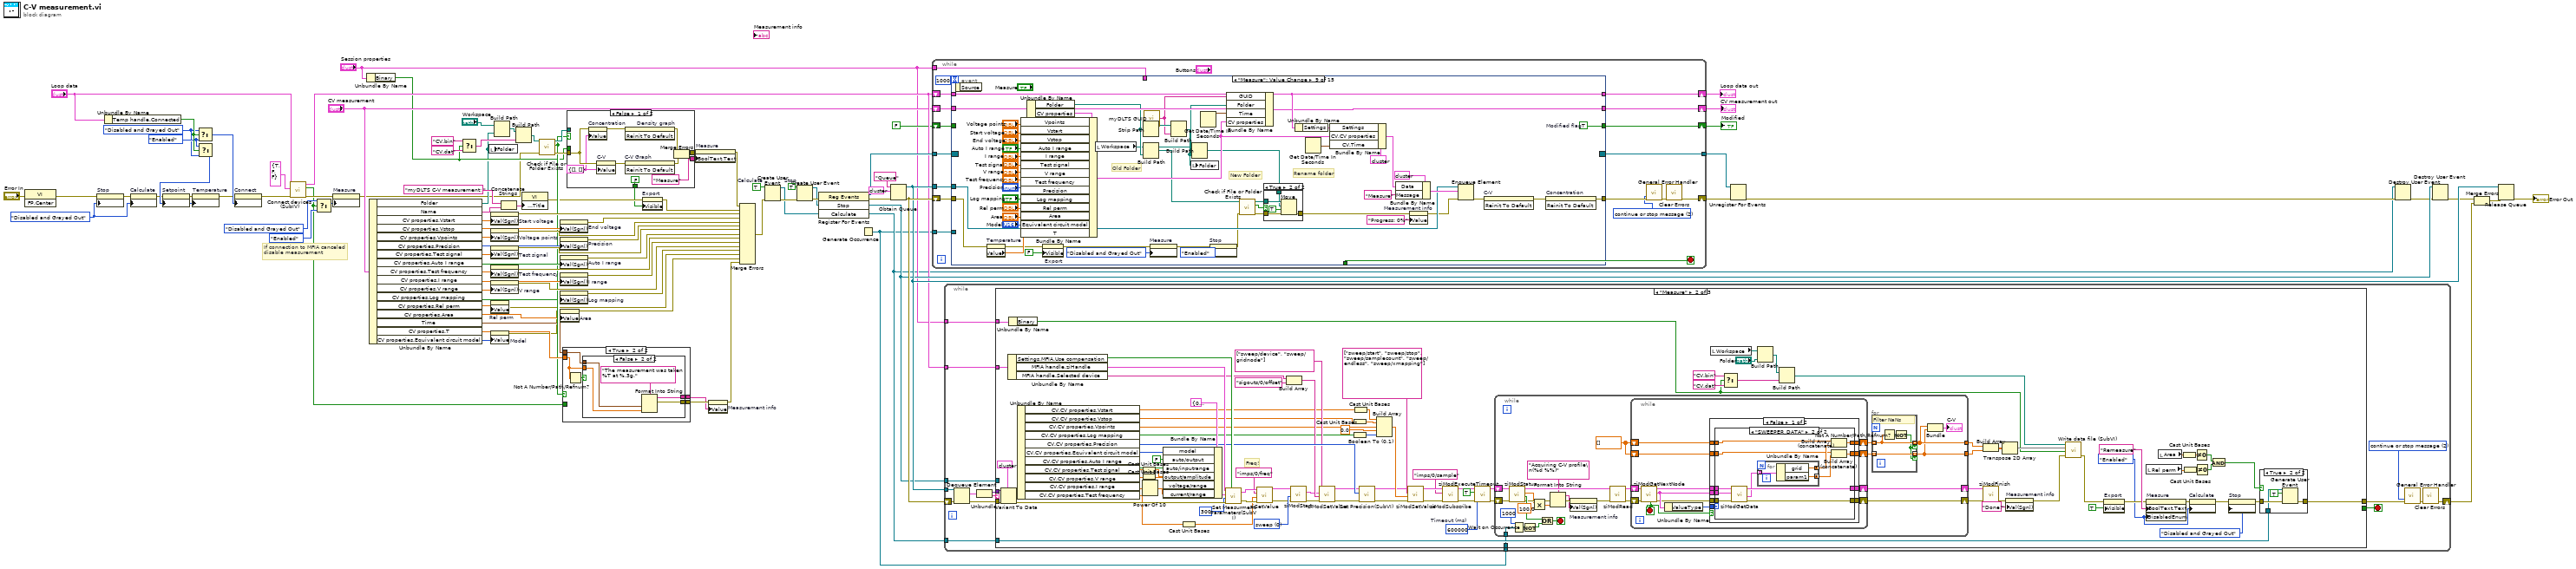
[diagram p0: block diagram]
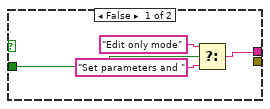
[diagram p2: hidden frame]
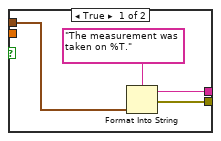
[diagram p3: hidden frame]
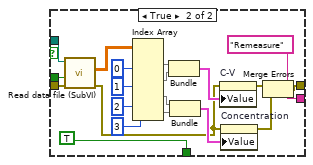
[diagram p4: hidden frame]
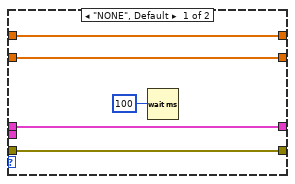
[diagram p6: hidden frame]
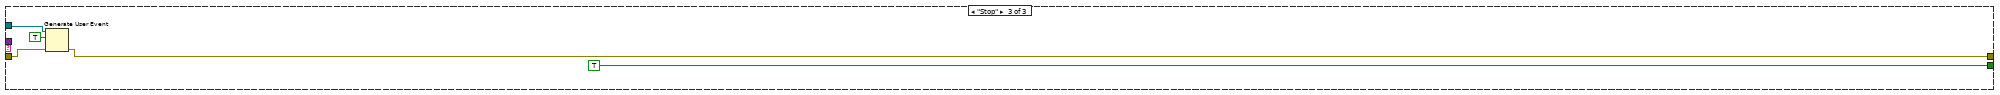
[diagram p9: hidden frame]
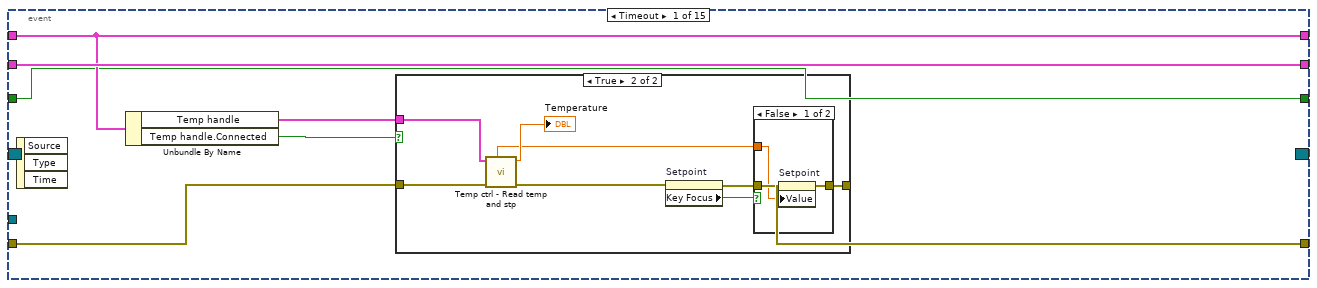
[diagram p10: hidden frame]
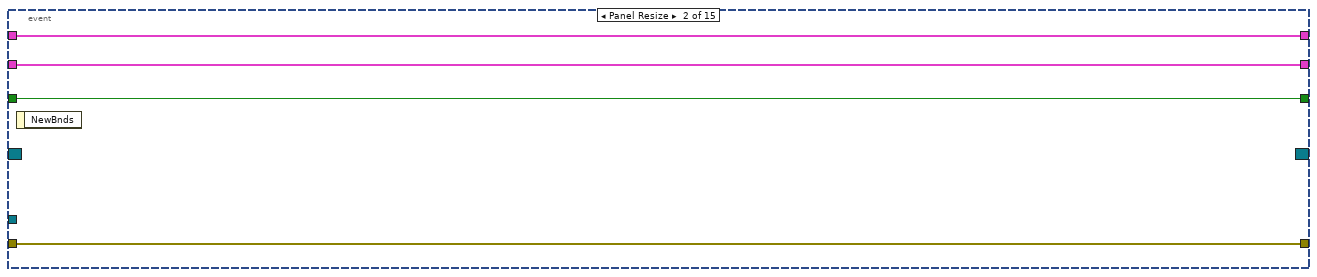
[diagram p13: hidden frame]
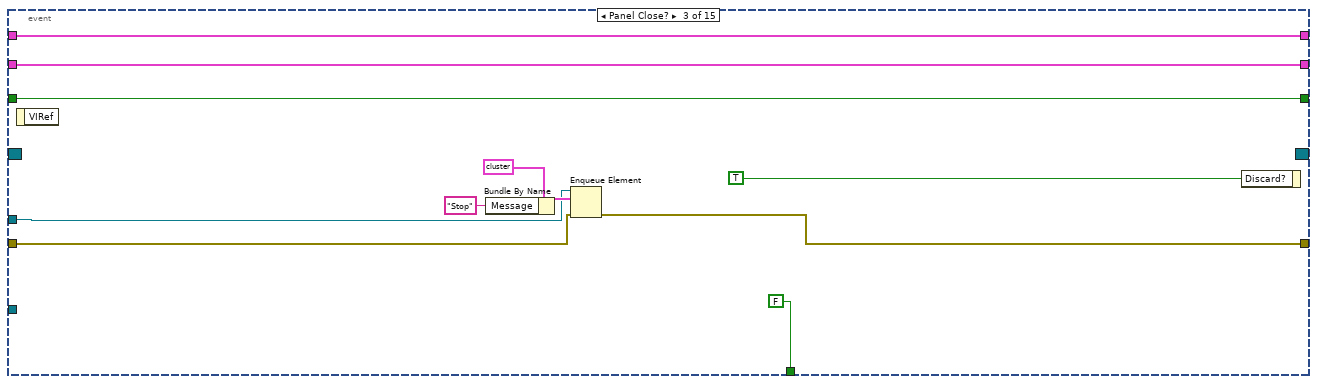
[diagram p14: hidden frame]
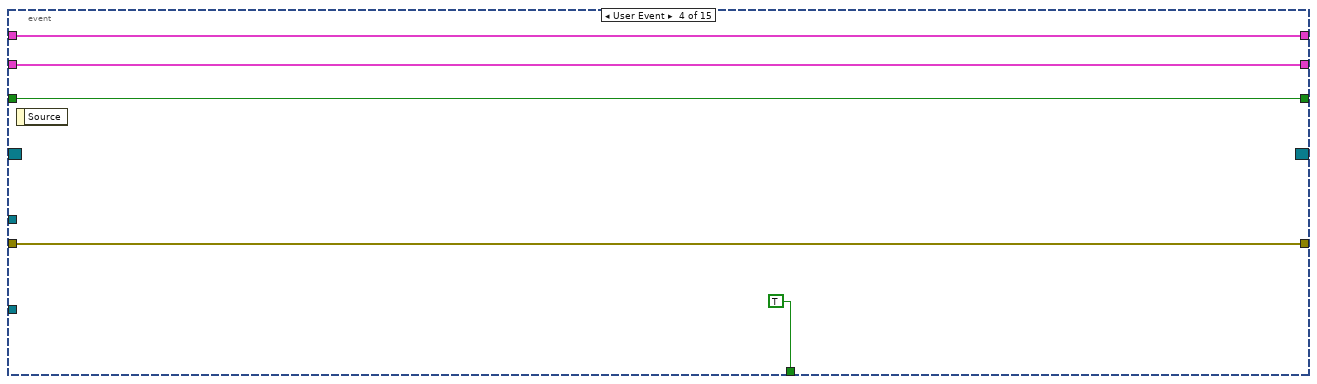
[diagram p15: hidden frame]
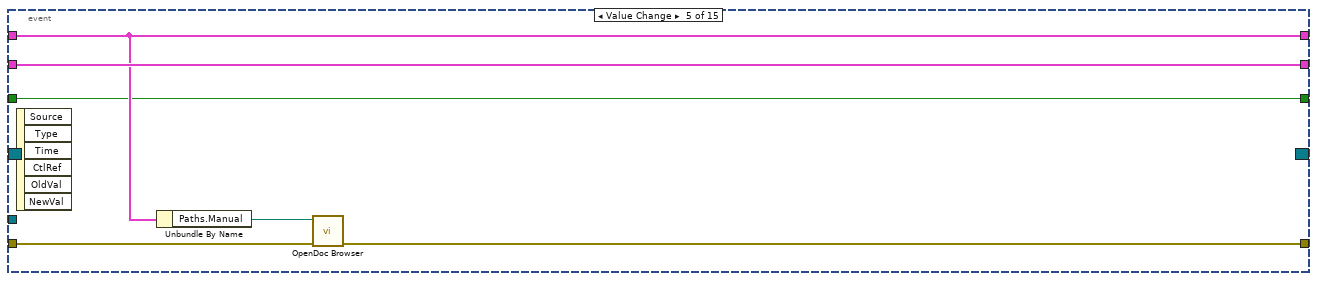
[diagram p16: hidden frame]
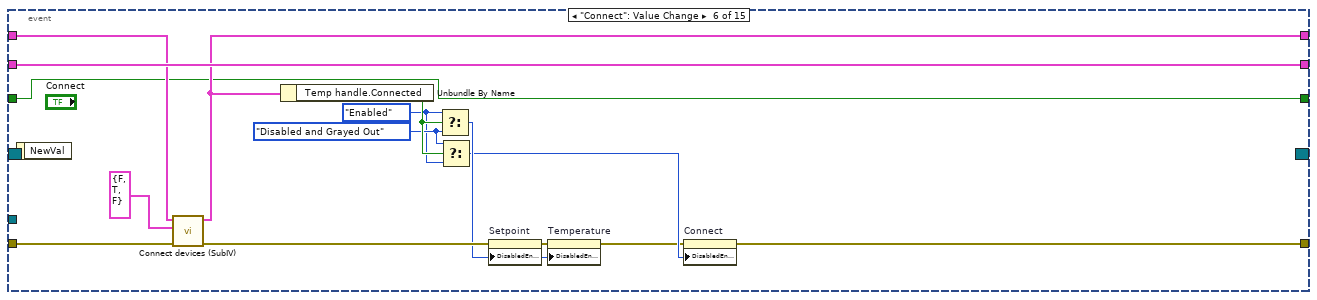
[diagram p17: hidden frame]
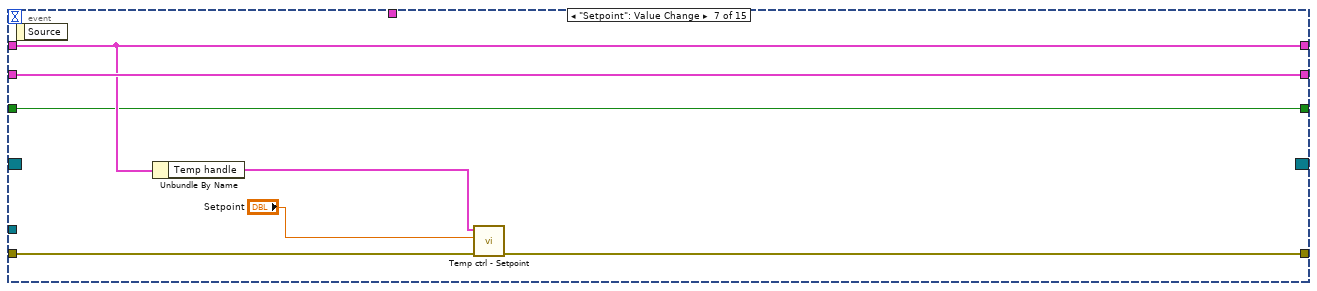
[diagram p18: hidden frame]
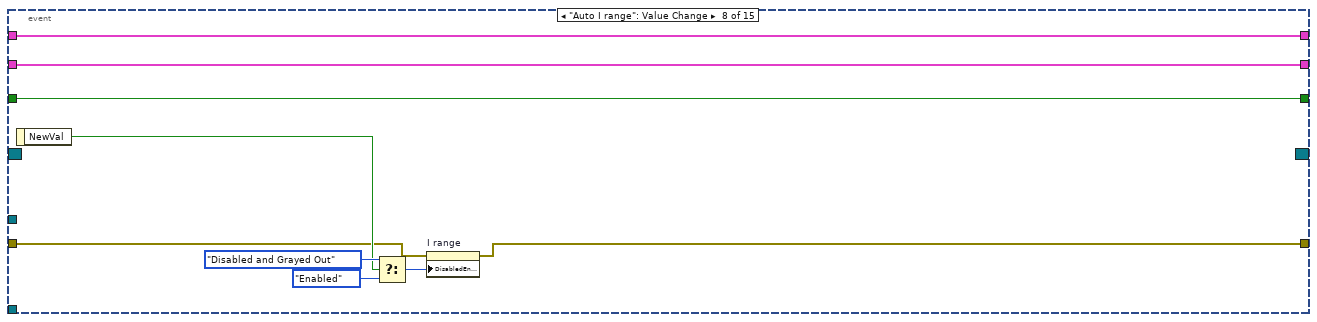
[diagram p19: hidden frame]
diagram:
  w4 = T24."Disabled and Grayed Out" ("Disabled")
  w21 = TRUE  # Calculate
  w80 = TRUE  # Stop
  w98 = T24."Enabled" ("f")
  w97 = T24."Disabled and Grayed Out" ("Disabled")
  # "If connection to MFIA canceled disable measurement"
  n1 = invoke class="VI" method="FP.Center"(error in="Error In") -> (error out=w5:errorcluster)  [unwired: 2 in, 2 out]
  n2 = property on="Stop" class="Bool"(error in=w5, "DisabledEnum"=w4) -> (error out=w6:errorcluster)  [unwired: 1 in, 1 out]
  n3 = Unbundle By Name("Loop data") -> ("Temp handle.Connected"=w99:bool)
  n4 = property on="Calculate" class="Bool"(error in=w6, "DisabledEnum"=w4) -> (error out=w17:errorcluster)  [unwired: 1 in, 1 out]
  n5 = Select(t=w97, s=w99, f=w98) -> (s? t:f=w79:T24)
  n6 = Select(t=w98, s=w99, f=w97) -> (s? t:f=w78:T24)
  n7 = property on="Setpoint" class="DigNum (strict)"(error in=w17, "DisabledEnum"=w78) -> (error out=w100:errorcluster)  [unwired: 1 in, 1 out]
  n8 = property on="Temperature" class="DigNum (strict)"(error in=w100, "DisabledEnum"=w78) -> (error out=w9:errorcluster)  [unwired: 1 in, 1 out]
  n9 = property on="Connect" class="Bool"(error in=w9, "DisabledEnum"=w79) -> (error out=w45:errorcluster)  [unwired: 1 in, 1 out]
  n10 = call "Connect devices (SubIV).vi"("Error In"=w45, "Devices"=T23 {"MFIA"=TRUE, "Temperature controller"=FALSE, "Source meter"=FALSE}, "Loop data in"="Loop data") -> ("Error Out"=w96:errorcluster, "Canceled"=w51:bool, "Loop data out"=w41:T3)  [unwired: 6 in]
  n11 = Select(t=T24."Disabled and Grayed Out" ("f"), s=w51, f=T24."Enabled") -> (s? t:f=w95:T24)
  n12 = property on="Measure" class="Bool"(error in=w96, "DisabledEnum"=w95) -> (error out=w1:errorcluster)  [unwired: 1 in, 1 out]
  n13 = Unbundle By Name("Session properties") -> ("Binary"=w25:bool)
  n14 = Unbundle By Name("CV measurement") -> ("Folder"=w8:path, "Name"=w43:string, "CV properties.Vstart"=w76:dbl[unit], "CV properties.Vstop"=w75:dbl[unit], "CV properties.Vpoints"=w77:dbl, "CV properties.Precision"=w74:enum16{"Low (Fast)", "Normal", "High (Slow)"}, "CV properties.Test signal"=w73:dbl[unit], "CV properties.Auto I range"=w72:bool, "CV properties.Test frequency"=w71:dbl[unit], "CV properties.I range"=w70:dbl, "CV properties.V range"=w69:dbl[unit], "CV properties.Log mapping"=w39:bool, "CV properties.Rel perm"=w16:dbl, "CV properties.Area"=w14:dbl[unit], "Time"=w13:timestamp, "CV properties.T"=w55:dbl[unit], "CV properties.Equivalent circuit model"=w3:u16)
  n15 = Select(t="CV.bin", s=w25, f="CV.dat") -> (s? t:f=w58:string)
  n16 = local write "Folder"(w8) -> ()
  n17 = property on="Start voltage" class="DigNum (strict)"("Val(Sgnl)"=w76) -> (error out=w68:errorcluster)  [unwired: 2 in, 1 out]
  n18 = property on="Voltage points" class="DigNum (strict)"("Val(Sgnl)"=w77) -> (error out=w66:errorcluster)  [unwired: 2 in, 1 out]
  n19 = property on="Test signal" class="DigNum (strict)"("Val(Sgnl)"=w73) -> (error out=w64:errorcluster)  [unwired: 2 in, 1 out]
  n20 = property on="Test frequency" class="DigNum (strict)"("Val(Sgnl)"=w71) -> (error out=w62:errorcluster)  [unwired: 2 in, 1 out]
  n21 = property on="V range" class="Ring (strict)"("Val(Sgnl)"=w69) -> (error out=w60:errorcluster)  [unwired: 2 in, 1 out]
  n22 = property on="Rel perm" class="DigNum (strict)"("Value"=w16) -> (error out=w15:errorcluster)  [unwired: 2 in, 1 out]
  n23 = property on="Model" class="Ring (strict)"("Value"=w3) -> (error out=w2:errorcluster)  [unwired: 2 in, 1 out]
  n24 = Build Path(base path="Workspace", name or relative path=w8) -> (appended path=w87:path)
  n25 = Concatenate Strings("myDLTS C-V measurement: " ("string"), w43) -> (w44:string)
  n26 = Build Path(base path=w87, name or relative path=w58) -> (appended path=w86:path)
  n27 = property class="VI"("Front Panel.Title"=w44) -> (error out=w28:errorcluster)  [unwired: 2 in, 1 out]
  n28 = call <vilib>:"Check if File or Folder Exists.vi"("error in (no error)"=w1, "path"=w86) -> ("error out"=w84:errorcluster, "file or folder exists?"=w54:bool, "dup path"=w85:path)  [unwired: 7 in]
  n29 = property on="End voltage" class="DigNum (strict)"("Val(Sgnl)"=w75) -> (error out=w67:errorcluster)  [unwired: 2 in, 1 out]
  n30 = property on="Precision" class="Enum (strict)"("Val(Sgnl)"=w74) -> (error out=w65:errorcluster)  [unwired: 2 in, 1 out]
  n31 = property on="Auto I range" class="Bool (strict)"("Val(Sgnl)"=w72) -> (error out=w63:errorcluster)  [unwired: 2 in, 1 out]
  n32 = property on="I range" class="Ring (strict)"("Val(Sgnl)"=w70) -> (error out=w61:errorcluster)  [unwired: 2 in, 1 out]
  n33 = property on="Log mapping" class="Bool (strict)"("Val(Sgnl)"=w39) -> (error out=w12:errorcluster)  [unwired: 2 in, 1 out]
  n34 = property on="Area" class="DigNum (strict)"(error in=w2, "Value"=w14) -> (error out=w11:errorcluster)  [unwired: 1 in, 1 out]
  n35 = case shown="True" w54 {
    tunnel: w13 -> [_ w110]
    tunnel: w55 -> [_ w108]
    tunnel: [_ w107] -> w53
    tunnel: [w104 w106] -> w52
    tunnel: w51 -> [w105 _]
    frame False {
      n36 = Select(t="Edit only mode", s=w105, f="Set parameters and ") -> (s? t:f=w104:string)
    }
    frame True {
      n37 = Not A Number/Path/Refnum?(number/path/refnum=w108) -> (NaN/Path/Refnum?=w109:bool)
      n38 = case shown="False" w109 {
        tunnel: w110 -> [w113 w118]
        tunnel: w108 -> [_ w115]
        tunnel: [w112 w117] -> w107
        tunnel: [w111 w116] -> w106
        frame True {
          n39 = Format Into String(format string="The measurement was taken on %T.", w113) -> (resulting string=w111:string, error out=w112:errorcluster)  [unwired: 2 in]
        }
        frame False {
          n40 = Format Into String(format string="The measurement was taken %T at %.3g.", w118, w115) -> (resulting string=w116:string, error out=w117:errorcluster)  [unwired: 2 in]
        }
      }
    }
  }
  n41 = case shown="False" w54 {
    tunnel: w25 -> [_ w148]
    tunnel: w85 -> [_ w147]
    tunnel: w84 -> [w121 w146]
    tunnel: [w125 w130] -> w35
    tunnel: ["Measure" ("Boolean Text.Text") "Remeasure" ("Boolean Text.Text")] -> w33
    tunnel: [FALSE TRUE] -> w26
    frame False {
      w120 = cluster{"2D data":dbl[], "2D data":dbl[]} {"2D data"=[], "2D data"=[]} ("C-V")
      n42 = property on="Concentration" class="XYGraph (strict)"(error in=w121, "Value"=w120) -> (error out=w123:errorcluster)  [unwired: 1 in, 1 out]
      n43 = property on="C-V" class="XYGraph (strict)"(error in=w121, "Value"=w120) -> (error out=w122:errorcluster)  [unwired: 1 in, 1 out]
      n44 = invoke on="Density graph" class="XYGraph (strict)" method="Reinit To Default"(error in=w123) -> (error out=w126:errorcluster)  [unwired: 2 in, 2 out]
      n45 = invoke on="C-V Graph" class="XYGraph (strict)" method="Reinit To Default"(error in=w122) -> (error out=w124:errorcluster)  [unwired: 2 in, 2 out]
      n46 = Merge Errors(w126, w124) -> (w125:errorcluster)
    }
    frame True {
      n47 = call "Read data file (SubVI).vi"("error in"=w146, "Binary"=w148, "file path in"=w147) -> ("error out"=w131:errorcluster, "2D data"=w145:dbl[][])  [unwired: 5 in, 2 out]
      n48 = Index Array(array=w145, index (col) #1=0 ("disabled index (col)"), index (col) #2=1 ("index (col)"), index (col) #3=2 ("index (col)"), index (col) #4=3 ("index (col)")) -> (element #1=w142:dbl[], element #2=w141:dbl[], element #3=w134:dbl[], element #4=w133:dbl[])  [unwired: 4 in]
      n49 = Bundle("2D data"=w142, "2D data"=w141) -> (w140:cluster{"2D data":dbl[], "2D data":dbl[]})  [unwired: 1 in]
      n50 = Bundle("2D data"=w134, "2D data"=w133) -> (w132:cluster{"2D data":dbl[], "2D data":dbl[]})  [unwired: 1 in]
      n51 = property on="C-V" class="XYGraph (strict)"(error in=w131, "Value"=w140) -> (error out=w139:errorcluster)  [unwired: 1 in, 1 out]
      n52 = property on="Concentration" class="XYGraph (strict)"(error in=w131, "Value"=w132) -> (error out=w129:errorcluster)  [unwired: 1 in, 1 out]
      n53 = Merge Errors(w139, w129) -> (w130:errorcluster)
    }
  }
  n54 = property on="Export" class="Bool"(error in=w28, "Visible"=w26) -> (error out=w27:errorcluster)  [unwired: 1 in, 1 out]
  n55 = property on="Measure" class="Bool"(error in=w35, "BoolText.Text"=w33) -> (error out=w34:errorcluster)  [unwired: 1 in, 1 out]
  n56 = property on="Measurement info" class="Str"(error in=w53, "Value"=w52) -> (error out=w38:errorcluster)  [unwired: 1 in, 1 out]
  n57 = Merge Errors(w34, w27, w68, w67, w66, w65, w64, w63, w62, w61, w60, w12, w15, w11, w38) -> (w23:errorcluster)
  n58 = Create User Event(user event datatype=w21, error in=w23) -> (user event=w18:refnum<user-event>, error out=w22:errorcluster)
  n59 = Create User Event(user event datatype=w80, error in=w22) -> (user event=w46:refnum<user-event>, error out=w81:errorcluster)
  n60 = register-events(error in=w81, w46, w18) -> (reference out=w82:refnum<event-registration>, error out=w83:errorcluster)  [unwired: 1 in]
  n61 = Generate Occurrence() -> (w7:refnum<k4>)
  n62 = Obtain Queue(name (unnamed)="Queue", element data type=cluster{"Data":variant, "Message":string} {"Data"=variant, "Message"=""}, error in (no error)=w83) -> (queue out=w47:refnum<queue>, error out=w88:errorcluster)  [unwired: 2 in, 1 out]
  n63 = while {
    shift-right: [w161] -> w91
    shift-left: w41 -> [w164]
    shift-right: [w162] -> w92
    shift-left: "CV measurement" -> [w163]
    shift-right: [w150] -> w50
    shift-left: w88 -> [w165]
    tunnel: w47 -> [w160]
    tunnel: w82 -> [w159]
    tunnel: [w158] -> w49
    shift-right: [w156] -> w36
    shift-left: FALSE -> [w157]
    tunnel: "Session properties" -> [w151]
    tunnel: w7 -> [w149]
    stop <- w166 stop-if-true
    w152 = T26 2 items=["no dialog", "OK message", "continue or stop message", "OK message + warnings", "continue/stop + warnings"] ("type of dialog (OK msg:1)")
    n64 = event shown="[8] \"Measure\": Value Change" {
      selector: w159 -> [_ _ _ _ _ _ _ _ _ _ _ _ _ _ _]
      dyn-events: [_ _ _ _ _ _ _ _ _ _ _ _ _ _ _] -> w158
      timeout: 1000 -> [_ _ _ _ _ _ _ _ _ _ _ _ _ _ _]
      tunnel: [_ _ FALSE TRUE _ _ _ _ _ _ _ _ _ _ _] -> w166
      tunnel: w165 -> [w172 w188 w193 w202 w212 w226 w231 w239 w280 w304 w322 w388 w414 w425 w457]
      tunnel: w164 -> [w171 w189 w198 w204 w209 w225 w233 w236 w296 w307 w316 w353 w416 w426 w459]
      tunnel: w163 -> [w173 w190 w199 w205 w210 w227 w234 w237 w277 w306 w315 w384 w417 w421 w451]
      tunnel: [w173 w190 w199 w205 w210 w227 w234 w237 w275 w306 w315 w376 w417 w422 w451] -> w162
      tunnel: [w171 w189 w198 w204 w209 w216 w233 w236 w296 w307 w316 w353 w416 w426 w459] -> w161
      tunnel: [w169 w188 w192 w202 w211 w217 w230 w238 w262 w304 w308 w365 w415 w424 w453] -> w154
      tunnel: w160 -> [_ _ w194 _ _ _ _ _ w291 _ _ _ _ _ _]
      tunnel: w157 -> [w168 w187 w191 w203 w208 w215 w232 w235 _ w305 w314 _ w418 w420 w460]
      tunnel: [w168 w187 w191 w203 w208 w215 w232 w235 w272 w305 w314 TRUE w418 w423 w460] -> w156
      tunnel: w151 -> [_ _ _ _ _ _ _ _ _ _ _ w352 _ _ w454]
      tunnel: w149 -> [_ _ _ _ _ _ _ _ _ w303 _ _ _ _ _]
      event Timeout {
        n65 = event-data() -> ()  [unwired: 1 in, 3 out]
        n66 = Unbundle By Name(w171) -> ("Temp handle"=w167:T5, "Temp handle.Connected"=w170:bool)
        n67 = case shown="True" w170 {
          tunnel: w172 -> [w174 w179]
          tunnel: [w174 w181] -> w169
          tunnel: w167 -> [_ w177]
          frame False {
          }
          frame True {
            n68 = call "Temp ctrl - Read temp and stp.vi"("Error In"=w179, "Temp handle"=w177) -> ("Error Out"=w178:errorcluster, "Sample temperature"=→"Temperature":dbl[unit], "Setpoint"=w175:dbl[unit])  [unwired: 2 in, 2 out]
            n69 = property on="Setpoint" class="DigNum (strict)"(error in=w178) -> (error out=w182:errorcluster, "Key Focus"=w180:bool)  [unwired: 1 in, 1 out]
            n70 = case shown="False" w180 {
              tunnel: w182 -> [w184 w186]
              tunnel: [w185 w186] -> w181
              tunnel: w175 -> [w183 _]
              frame False {
                n71 = property on="Setpoint" class="DigNum (strict)"(error in=w184, "Value"=w183) -> (error out=w185:errorcluster)  [unwired: 1 in, 1 out]
              }
              frame True {
              }
            }
          }
        }
      }
      event Panel Resize {
        n72 = event-data() -> ()  [unwired: 1 in, 1 out]
      }
      event Panel Close? {
        n73 = event-data() -> ()  [unwired: 1 in, 1 out]
        n74 = Bundle By Name(cluster=cluster{"Data":variant, "Message":string} {"Data"=variant, "Message"=""}, "Message"="Stop") -> (w196:cluster{"Data":variant, "Message":string})
        n75 = Enqueue Element(queue=w194, element=w196, error in (no error)=w193) -> (error out=w192:errorcluster)  [unwired: 1 in, 2 out]
        n76 = event-data("Discard?"=TRUE) -> ()  [unwired: 1 in, 1 out]
      }
      event User Event {
        n77 = event-data() -> ()  [unwired: 1 in, 1 out]
      }
      event "Buttons.Help": Value Change {
        n78 = event-data() -> ()  [unwired: 1 in, 6 out]
        n79 = Unbundle By Name(w209) -> ("Paths.Manual"=w207:path)
        n80 = call "OpenDoc Browser.vi"("error in (no error)"=w212, "File"=w207) -> ("error out"=w211:errorcluster)  [unwired: 9 in]
      }
      event "Connect": Value Change {
        w223 = T24."Disabled and Grayed Out" ("f")
        w222 = T24."Enabled" ("Disabled")
        n81 = event-data() -> ()  [unwired: 1 in, 1 out]
        n82 = call "Connect devices (SubIV).vi"("Error In"=w226, "Devices"=T23 {"MFIA"=FALSE, "Temperature controller"=TRUE, "Source meter"=FALSE}, "Loop data in"=w225) -> ("Error Out"=w221:errorcluster, "Loop data out"=w216:T3)  [unwired: 6 in, 1 out]
        n83 = Unbundle By Name(w216) -> ("Temp handle.Connected"=w224:bool)
        n84 = Select(t=w222, s=w224, f=w223) -> (s? t:f=w219:T24)
        n85 = Select(t=w223, s=w224, f=w222) -> (s? t:f=w218:T24)
        n86 = property on="Setpoint" class="DigNum (strict)"(error in=w221, "DisabledEnum"=w219) -> (error out=w220:errorcluster)  [unwired: 1 in, 1 out]
        n87 = property on="Temperature" class="DigNum (strict)"(error in=w220, "DisabledEnum"=w219) -> (error out=w213:errorcluster)  [unwired: 1 in, 1 out]
        n88 = property on="Connect" class="Bool"(error in=w213, "DisabledEnum"=w218) -> (error out=w217:errorcluster)  [unwired: 1 in, 1 out]
      }
      event "Setpoint": Value Change {
        n89 = event-data() -> ()  [unwired: 1 in, 1 out]
        n90 = Unbundle By Name(w233) -> ("Temp handle"=w229:T5)
        n91 = call "Temp ctrl - Setpoint.vi"("Error In"=w231, "Setpoint"="Setpoint", "Temp handle"=w229) -> ("Error Out"=w230:errorcluster)  [unwired: 8 in]
      }
      event "Auto I range": Value Change {
        n92 = event-data() -> ("NewVal"=w240:bool)  [unwired: 1 in]
        n93 = Select(t=T24."Disabled and Grayed Out", s=w240, f=T24."Enabled") -> (s? t:f=w243:T24)
        n94 = property on="I range" class="Ring (strict)"(error in=w239, "DisabledEnum"=w243) -> (error out=w238:errorcluster)  [unwired: 1 in, 1 out]
      }
      event "Measure": Value Change {
        w272 = TRUE  # Modified flag
        # "Rename folder"
        # "New Folder"
        # "Old Folder"
        n95 = event-data() -> ()  [unwired: 1 in, 1 out]
        n96 = property on="Temperature" class="DigNum (strict)"(error in=w280) -> (error out=w261:errorcluster, "Value"=w273:dbl[unit])  [unwired: 1 in, 1 out]
        n97 = Unbundle By Name(w277) -> ("Folder"=w258:path, "CV properties"=w290:T15)
        n98 = Bundle By Name(cluster=w290, "Vpoints"="Voltage points", "Vstart"="Start voltage", "Vstop"="End voltage", "Auto I range"="Auto I range", "I range"="I range", "Test signal"="Test signal", "V range"="V range", "Test frequency"="Test frequency", "Precision"="Precision", "Log mapping"="Log mapping", "Rel perm"="Rel perm", "Area"="Area", "Equivalent circuit model"="Model", "T"=w273) -> (w276:T15)
        n99 = property on="Export" class="Bool"(error in=w261, "Visible"=FALSE) -> (error out=w268:errorcluster)  [unwired: 1 in, 1 out]
        n100 = local read "Workspace"() -> (w252:path)
        n101 = Strip Path(path=w258) -> (stripped path=w259:path)  [unwired: 1 out]
        n102 = Build Path(base path=w252, name or relative path=w258) -> (appended path=w250:path)
        n103 = call "myDLTS GUID.vi"() -> ("GUID"=w248:string)  [unwired: 1 in]
        n104 = property on="Measure" class="Bool"(error in=w268, "DisabledEnum"=T24."Disabled and Grayed Out" ("Disabled")) -> (error out=w247:errorcluster)  [unwired: 1 in, 1 out]
        n105 = Build Path(base path=w259, name or relative path=w248) -> (appended path=w257:path)
        n106 = local write "Folder"(w257) -> ()
        n107 = Build Path(base path=w252, name or relative path=w257) -> (appended path=w253:path)
        n108 = Get Date/Time In Seconds() -> (seconds since 1Jan1904=w249:timestamp)
        n109 = property on="Stop" class="Bool"(error in=w247, "DisabledEnum"=T24."Enabled" ("Disabled")) -> (error out=w246:errorcluster)  [unwired: 1 in, 1 out]
        n110 = Bundle By Name(cluster=w277, "GUID"=w248, "Folder"=w257, "Time"=w249, "CV properties"=w276) -> (w275:T22)
        n111 = call <vilib>:"Check if File or Folder Exists.vi"("error in (no error)"=w246, "path"=w250) -> ("error out"=w256:errorcluster, "file or folder exists?"=w254:bool, "dup path"=w255:path)  [unwired: 7 in]
        n112 = case shown="True" w254 {
          tunnel: w255 -> [_ w301]
          tunnel: w253 -> [_ w300]
          tunnel: w256 -> [w297 w299]
          tunnel: [w297 w298] -> w251
          frame False {
          }
          frame True {
            n113 = Move(source path=w301, error in=w299, 9:TRUE ("overwrite (F)"), 10:w300) -> (error out=w298:errorcluster)  [unwired: 1 in, 2 out]
          }
        }
        n114 = Unbundle By Name(w296) -> ("Settings"=w295:T9)
        n115 = Get Date/Time In Seconds() -> (seconds since 1Jan1904=w279:timestamp)
        n116 = Bundle By Name(cluster=cluster{"Settings":T9, "CV":T22} {"Settings"={"MFIA"={"Address"="", "Use compensation"=TRUE, "Shut down gracefully"=FALSE}, "Temp ctrl"={"Gain (P)"=0.0, "Reset (I)"=0.0, "Rate (D)"=0.0, "Stabilization rate"=0.0, "Stabilization delta"=0.0, "Type"=enum."Lake Shore 325", "Custom temp ctrl"={"VISA resource name"=""}, "Lakeshore 325"={"VISA name"="", "Loop"=0, "Heater Range"=1, "Heater Resistance"=0, "Sample sensor"=0, "Fast sensor"=0, "Slow sensor"=0}, "Lakeshore 331"={"VISA name"="", "Loop"=1, "Heater Range"=0, "Sample sensor"=0, "Fast sensor"=0, "Slow sensor"=0}, "Lakeshore 332"={"VISA name"="", "Loop"=1, "Heater Range"=0, "Sample sensor"=0, "Fast sensor"=0, "Slow sensor"=0}, "Lakeshore 335"={"VISA name"="", "Loop"=1, "Sample sensor"=0, "Fast sensor"=0, "Slow sensor"=0, "Heater Range"=0, "Output mode"=enum."Off"}, "Lakeshore 336"={"VISA name"="", "Loop"=1, "Output mode"=enum."Off", "Max current"=1.0, "Heater resistance"=1, "Sample sensor"=1, "Slow sensor"=1, "Fast sensor"=1}}, "Source-meter"={"Type"=enum."Custom", "Custom source-meter"={"VISA resource name"=""}, "Keithley 2600"={"VISA name"="", "Ignore ID Query"=FALSE, "SMU"=enum."Channel A"}, "Keithley 2400 Series"={"VISA name"="", "Ignore ID Query"=FALSE}}, "Other"={"Enable OriginLab"=FALSE, "Reader mode"=FALSE, "Auto-save"=FALSE}, "Defaults"={"IV properties"={"T"=0.0, "Vstart"=-0.5, "Vstop"=0.5, "Vpoints"=10.0, "Settling"=0.01, "I limit"=0.1, "Log mapping"=FALSE, "Averaging"=0.0}, "CV properties"={"T"=0.0, "Vstart"=-0.5, "Vstop"=0.5, "Vpoints"=10.0, "Precision"=enum."Normal", "Test signal"=0.01, "Auto I range"=FALSE, "Test frequency"=100000.0, "I range"=-2.0, "V range"=10.0, "Log mapping"=FALSE, "Rel perm"=0.0, "Area"=0.0, "Equivalent circuit model"=0}, "DLTS properties"={"Tstart"=0.0, "Instant start"=FALSE, "Tstop"=0.0, "T rate"=0.0, "Test signal"=0.0, "Test frequency"=0.0, "Bandwidth"=0.0, "Averaging"=0.0, "Vbias"=0.0, "Vpulse"=0.0, "pulse length"=0.0, "Pulse 2"=FALSE, "Vpulse 2"=0.0, "pulse length 2"=0.0, "I range"=-2.0, "V range"=10.0, "Emission rate"=[], "Sampling rate"=0.0, "Acq. delay"=0.0, "Filter order"=0, "Equivalent circuit model"=0}, "LDLTS properties"={"T"=0.0, "Test signal"=0.0, "Test frequency"=0.0, "Bandwidth"=0.0, "Averaging"=0.0, "Vbias"=0.0, "Vpulse"=0.0, "pulse length"=0.0, "Pulse 2"=FALSE, "Vpulse 2"=0.0, "pulse length 2"=0.0, "I range"=-2.0, "V range"=10.0, "Sampling rate"=0.0, "Acq. delay"=0.0, "Sampling time"=0.0, "Filter order"=0, "Equivalent circuit model"=0}}}, "CV"={"Name"="", "Comment"="", "Time"=timestamp(0 s since 1904-01-01), "Folder"=path "", "CV properties"={"T"=0.0, "Vstart"=0.0, "Vstop"=0.0, "Vpoints"=0.0, "Precision"=enum."Low (Fast)", "Test signal"=0.0, "Auto I range"=FALSE, "Test frequency"=0.0, "I range"=0.0, "V range"=0.0, "Log mapping"=FALSE, "Rel perm"=0.0, "Area"=0.0, "Equivalent circuit model"=0}, "GUID"=""}}, "Settings"=w295, "CV.CV properties"=w276, "CV.Time"=w279) -> (w292:cluster{"Settings":T9, "CV":T22})
        n117 = Bundle By Name(cluster=cluster{"Data":variant, "Message":string} {"Data"=variant, "Message"=""}, "Data"=w292, "Message"="Measure") -> (w293:cluster{"Data":variant, "Message":string})
        n118 = property on="Measurement info" class="Str"(error in=w251, "Value"="Progress: 0%" ("Measurement info")) -> (error out=w271:errorcluster)  [unwired: 1 in, 1 out]
        n119 = Enqueue Element(queue=w291, element=w293, error in (no error)=w271) -> (error out=w264:errorcluster)  [unwired: 1 in, 2 out]
        n120 = invoke on="C-V" class="XYGraph (strict)" method="Reinit To Default"(error in=w264) -> (error out=w263:errorcluster)  [unwired: 2 in, 2 out]
        n121 = invoke on="Concentration" class="XYGraph (strict)" method="Reinit To Default"(error in=w263) -> (error out=w262:errorcluster)  [unwired: 2 in, 2 out]
      }
      event "Stop": Value Change {
        n122 = event-data() -> ()  [unwired: 1 in, 1 out]
        n123 = Set Occurrence(w303) -> ()
      }
      event "Start voltage", "End voltage", "Test signal", "V range": Value Change {
        # "Coerce voltages based on test signal snd V range"
        n124 = event-data() -> ()  [unwired: 1 in, 1 out]
        n125 = property on="Test signal" class="DigNum (strict)"(error in=w322) -> (error out=w317:errorcluster, "Value"=w321:dbl[unit])  [unwired: 1 in, 1 out]
        n126 = Multiply(x=w321, y=1.42) -> (x*y=w318:dbl[unit])
        n127 = property on="V range" class="Ring (strict)"(error in=w317) -> (error out=w313:errorcluster, "Value"=w319:dbl[unit])  [unwired: 1 in, 1 out]
        n128 = control-ref of="Start voltage"() -> (w311:refnum<vi>)
        n129 = control-ref of="End voltage"() -> (w310:refnum<vi>)
        n130 = Subtract(x=w319, y=w318) -> (x-y=w312:dbl[unit])
        n131 = Build Array(w311, w310) -> (w309:refnum<vi>[])
        n132 = for {
          tunnel: w313 -> [w327]
          tunnel: w312 -> [w326]
          tunnel: w309 -> [w324] mode=indexing
          tunnel: [w323] -> w308
          n133 = property on="Property Node" class="DigNum (strict)"(reference=w324, error in=w327) -> (reference out=w325:refnum<vi>, error out=w329:errorcluster, "Value"=w328:dbl[unit])
          n134 = Negate(x=w326) -> (-x=w332:dbl[unit])
          n135 = In Range and Coerce(upper limit=w326, x=w328, lower limit=w332) -> (coerced(x)=w330:dbl[unit], In Range?=w331:bool)
          n136 = case shown="False" w331 {
            tunnel: w330 -> [w335 _]
            tunnel: w329 -> [w336 w337]
            tunnel: [w334 w337] -> w323
            tunnel: w325 -> [w333 _]
            frame False {
              # "Coerce"
              n137 = property on="Property Node" class="DigNum (strict)"(reference=w333, error in=w336, "Value"=w335) -> (error out=w334:errorcluster)  [unwired: 1 out]
            }
            frame True {
              # "In Range"
            }
          }
        }
      }
      event User Event; "Calculate": Value Change {
        w338 = sgl nan ("new element/subarray")
        w339 = nan
        w340 = 0 ("index")
        w377 = u16 0 items=["2nd Order Central", "4th Order Central", "Forward", "Backward"] ("method")
        w386 = T27 25 items=["LabVIEW UI"=0, "ActiveX"=1, "User Event"=25] ("Source")
        n138 = event-data() -> ("Source"=w387:T27)  [unwired: 1 in]
        n139 = local read "C-V"() -> (w383:cluster{"2D data":dbl[], "2D data":dbl[]})
        n140 = Equal?(x=w387, y=w386) -> (x = y?=w385:bool)
        n141 = case shown="False" w385 {
          tunnel: w384 -> [w399 w400]
          tunnel: [w398 w400] -> w376
          frame False {
            n142 = local read "Rel perm"() -> (w397:dbl)
            n143 = local read "Area"() -> (w396:dbl[unit])
            n144 = Bundle By Name(cluster=w399, "CV properties.Rel perm"=w397, "CV properties.Area"=w396) -> (w398:T22)
          }
          frame True {
          }
        }
        n145 = Unbundle(w383) -> ("2D data"=w364:dbl[], "2D data"=w363:dbl[])
        n146 = Index Array(array=w364, index #1=1 ("index"), index #2=0 ("index")) -> (element #1=w381:dbl, element #2=w382:dbl)
        n147 = property on="Calculate" class="Bool"(error in=w388, "DisabledEnum"=T24."Disabled and Grayed Out" ("Disabled")) -> (error out=w350:errorcluster)  [unwired: 1 in, 1 out]
        n148 = Subtract(x=w381, y=w382) -> (x-y=w378:dbl)
        n149 = call <vilib>:"Derivative x(t).vi"("method"=w377, "dt"=w378, "X"=w363) -> ("dX/dt"=w372:dbl[])  [unwired: 7 in, 1 out]
        n150 = Unbundle By Name(w352) -> ("Binary"=w351:bool)
        n151 = Unbundle By Name(w376) -> ("CV properties.Rel perm"=w375:dbl, "CV properties.Area"=w374:dbl[unit], "Folder"=w354:path)
        n152 = Cast Unit Bases(0:w374) -> (2:w373:dbl)  [unwired: 1 in]
        n153 = for {
          tunnel: w375 -> [w395]
          tunnel: w373 -> [w394]
          tunnel: w363 -> [w393] mode=indexing
          tunnel: w372 -> [w392] mode=indexing
          tunnel: [w391] -> w371 mode=indexing
          tunnel: [w390] -> w343 mode=indexing
          n154 = formula code="float32 x = A*eps*8.85e-12/C;\nfloat32 N = (-C*C*C)/(A*A*eps*8.85e-12*1.6e-19*Cprim);\nN = abs(N);"("eps"=w395, "A"=w394, "C"=w393, "Cprim"=w392) -> ("x"=w391:sgl, "N"=w390:sgl)
        }
        n155 = Select(t="CV.bin", s=w351, f="CV.dat") -> (s? t:f=w357:string)
        n156 = local read "Workspace"() -> (w355:path)
        n157 = Build Path(base path=w355, name or relative path=w354) -> (appended path=w360:path)
        n158 = Build Path(base path=w360, name or relative path=w357) -> (appended path=w356:path)
        n159 = node(w371) -> (w362:sgl[unit][])
        n160 = node(w343) -> (w370:sgl[unit][])
        n161 = Array Size(array=w343) -> (size(s)=w342:i32)
        n162 = Cast Unit Bases(0:w362) -> (2:w347:sgl[])  [unwired: 1 in]
        n163 = Decrement(x=w342) -> (x-1=w341:i32)
        n164 = node(w370) -> (w361:sgl[])
        n165 = Cast Unit Bases(0:w361) -> (2:w345:sgl[])  [unwired: 1 in]
        n166 = Replace Array Subset(array=w345, new element=w339, index=w340) -> (w344:sgl[])
        n167 = Replace Array Subset(array=w347, new element=w338, index=w340) -> (w346:sgl[])
        n168 = Replace Array Subset(array=w346, new element=w338, index=w341) -> (w349:sgl[])
        n169 = Replace Array Subset(array=w344, new element=w339, index=w341) -> (w348:sgl[])
        n170 = Bundle(w349, w348) -> (→"Concentration":cluster{sgl[], sgl[]})  [unwired: 1 in]
        n171 = Build Array(w364, w363, w349, w348) -> (w367:dbl[][])
        n172 = Transpose 2D Array(2D array=w367) -> (transposed array=w366:dbl[][])
        n173 = call "Write data file (SubVI).vi"("error in"=w350, "Binary"=w351, "2D data"=w366, "file path in"=w356) -> ("error out"=w365:errorcluster)  [unwired: 6 in, 1 out]
      }
      event "Rel perm", "Area": Value Change {
        n174 = event-data() -> ()  [unwired: 1 in, 1 out]
        n175 = local read "Rel perm"() -> (w411:dbl)
        n176 = local read "Area"() -> (w410:dbl[unit])
        n177 = local read "C-V"() -> (w413:cluster{"2D data":dbl[], "2D data":dbl[]})
        n178 = Cast Unit Bases(0:w411) -> (2:w409:dbl)  [unwired: 1 in]
        n179 = Cast Unit Bases(0:w410) -> (2:w408:dbl)  [unwired: 1 in]
        n180 = Not Equal To 0?(x=w409) -> (x != 0?=w407:bool)
        n181 = Not Equal To 0?(x=w408) -> (x != 0?=w406:bool)
        n182 = Not Equal?(x=w413, y=cluster{"2D data":dbl[], "2D data":dbl[]} {"2D data"=[], "2D data"=[]}) -> (x != y?=w405:bool)
        n183 = Compound Arithmetic op=AND(w407, w406, w405) -> (w404:bool)
        n184 = Select(t=T24."Enabled" ("Disabled"), s=w404, f=T24."Disabled and Grayed Out") -> (s? t:f=w402:T24)
        n185 = property on="Calculate" class="Bool"(error in=w414, "DisabledEnum"=w402) -> (error out=w415:errorcluster)  [unwired: 1 in, 1 out]
      }
      event "Buttons.Information": Value Change {
        n186 = event-data() -> ("NewVal"=w419:bool)  [unwired: 1 in]
        n187 = case shown="True" w419 {
          tunnel: w421 -> [w428 w435]
          tunnel: w425 -> [w427 w438]
          tunnel: [w427 w436] -> w424
          tunnel: [w428 w434] -> w422
          tunnel: w420 -> [w429 w433]
          tunnel: [w429 w432] -> w423
          frame False {
          }
          frame True {
            n188 = Unbundle By Name(w435) -> ("Name"=w440:string, "Comment"=w439:string)
            n189 = call "Measurement renamer.vi"("error in (no error)"=w438, "Comment In"=w439, "Measurement name In"=w440) -> ("error out"=w436:errorcluster, "Canceled"=w437:bool, "Comment Out"=w430:string, "Measurement name Out"=w431:string)  [unwired: 1 in]
            n190 = case shown="False" w437 {
              tunnel: w435 -> [w444 w447]
              tunnel: [w443 w447] -> w434
              tunnel: w433 -> [_ w446]
              tunnel: [TRUE w446] -> w432
              tunnel: w431 -> [w442 _]
              tunnel: w430 -> [w441 _]
              frame False {
                n191 = Bundle By Name(cluster=w444, "Name"=w442, "Comment"=w441) -> (w443:T22)
              }
              frame True {
              }
            }
          }
        }
      }
      event "Buttons.Export": Value Change {
        n192 = event-data() -> ()  [unwired: 1 in, 1 out]
        n193 = Unbundle By Name(w459) -> ("Settings.Other.Enable OriginLab"=w458:bool)
        n194 = local read "Workspace"() -> (w455:path)
        n195 = Bundle By Name(cluster=T25 {"Clipboard"=TRUE, "dat"=TRUE, "iso"=FALSE, "Origin"=FALSE, "Excel"=FALSE} ("Available options"), "Origin"=w458) -> (w448:T25)
        n196 = call "Export dialog.vi"("error in (no error)"=w457, "Available options"=w448) -> ("error out"=w452:errorcluster, "Option"=w456:T28)  [unwired: 7 in, 1 out]
        n197 = case shown="\"Clipboard\"" w456 {
          tunnel: w455 -> [_ w464 w468 w475]
          tunnel: w454 -> [_ _ _ w474]
          tunnel: w451 -> [_ w463 w467 w473]
          tunnel: [w461 w466 w470 w472] -> w453
          tunnel: w452 -> [w461 w465 w469 w471]
          tunnel: "myDLTS file path" -> [_ w462 _ _]
          frame "Canceled", Default {
          }
          frame "Dat" {
            n198 = call-poly "Export single dat - cluster.vi"(".myDLTS file path"=w462, "Error In"=w465, "Workspace"=w464, "CV measurement"=w463) -> ("Error Out"=w466:errorcluster)  [unwired: 4 in]
          }
          frame "Clipboard" {
            n199 = call-poly "Export single clipboard - cluster.vi"("Error In"=w469, "Workspace"=w468, "CV measurement"=w467) -> ("Error Out"=w470:errorcluster)  [unwired: 5 in]
          }
          frame "Origin" {
            n200 = call-poly "Export Origin.vi"("Error In"=w471, "Workspace"=w475, "Session properties"=w474, "CV measurement"=w473) -> ("Error Out"=w472:errorcluster)  [unwired: 7 in]
          }
        }
      }
    }
    n201 = call <vilib>:"General Error Handler.vi"("type of dialog (OK msg:1)"=w152, "error in (no error)"=w154) -> ("error out"=w153:errorcluster)  [unwired: 9 in, 4 out]
    n202 = call <vilib>:"Clear Errors.vi"("error in (no error)"=w153) -> ("error out"=w150:errorcluster)  [unwired: 5 in, 1 out]
  }
  "Loop data out" <- w91
  "CV measurement out" <- w92
  "Modified" <- w36
  n203 = while {
    tunnel: w47 -> [w490]
    shift-right: [w478] -> w29
    shift-left: w88 -> [w491]
    tunnel: w46 -> [w485]
    tunnel: w41 -> [w483]
    tunnel: "Session properties" -> [w479]
    tunnel: w18 -> [w477]
    tunnel: w7 -> [w476]
    stop <- w484 stop-if-true
    w480 = T26 2 items=["no dialog", "OK message", "continue or stop message", "OK message + warnings", "continue/stop + warnings"] ("type of dialog (OK msg:1)")
    n204 = Dequeue Element(queue=w490, error in (no error)=w491) -> (element=w489:cluster{"Data":variant, "Message":string}, error out=w486:errorcluster)  [unwired: 1 in, 2 out]
    n205 = Unbundle(w489) -> ("Data"=w487:variant, "Message"=w488:string)
    n206 = case shown="\"Measure\"" w488 {
      tunnel: w487 -> [_ w586 _]
      tunnel: w486 -> [w492 w587 w675]
      tunnel: w485 -> [_ _ w674]
      tunnel: [w492 w510 w672] -> w482
      tunnel: [_ _ TRUE] -> w484
      tunnel: w483 -> [_ w577 _]
      tunnel: w479 -> [_ w523 _]
      tunnel: w477 -> [_ w509 _]
      tunnel: w476 -> [_ w498 _]
      frame "", Default {
      }
      frame "Measure" {
        w507 = u32 600000  # Timeout (ms)
        w518 = T24."Enabled" ("Disabled")
        w572 = T30 0 items=["sweep", "scopeModule", "dataAcquisitionModule", "pidAdvisor", "awgModule", "impedanceModule", "multiDeviceSyncModule", "zoomFFT", "trigger", "deviceSettings", "record", "precompensationAdvisor"] ("module Id")
        # "Freq!"
        n207 = Variant To Data(error in=w587, type=cluster{"Settings":T9, "CV":T22} {"Settings"={"MFIA"={"Address"="", "Use compensation"=TRUE, "Shut down gracefully"=FALSE}, "Temp ctrl"={"Gain (P)"=0.0, "Reset (I)"=0.0, "Rate (D)"=0.0, "Stabilization rate"=0.0, "Stabilization delta"=0.0, "Type"=enum."Lake Shore 325", "Custom temp ctrl"={"VISA resource name"=""}, "Lakeshore 325"={"VISA name"="", "Loop"=0, "Heater Range"=1, "Heater Resistance"=0, "Sample sensor"=0, "Fast sensor"=0, "Slow sensor"=0}, "Lakeshore 331"={"VISA name"="", "Loop"=1, "Heater Range"=0, "Sample sensor"=0, "Fast sensor"=0, "Slow sensor"=0}, "Lakeshore 332"={"VISA name"="", "Loop"=1, "Heater Range"=0, "Sample sensor"=0, "Fast sensor"=0, "Slow sensor"=0}, "Lakeshore 335"={"VISA name"="", "Loop"=1, "Sample sensor"=0, "Fast sensor"=0, "Slow sensor"=0, "Heater Range"=0, "Output mode"=enum."Off"}, "Lakeshore 336"={"VISA name"="", "Loop"=1, "Output mode"=enum."Off", "Max current"=1.0, "Heater resistance"=1, "Sample sensor"=1, "Slow sensor"=1, "Fast sensor"=1}}, "Source-meter"={"Type"=enum."Custom", "Custom source-meter"={"VISA resource name"=""}, "Keithley 2600"={"VISA name"="", "Ignore ID Query"=FALSE, "SMU"=enum."Channel A"}, "Keithley 2400 Series"={"VISA name"="", "Ignore ID Query"=FALSE}}, "Other"={"Enable OriginLab"=FALSE, "Reader mode"=FALSE, "Auto-save"=FALSE}, "Defaults"={"IV properties"={"T"=0.0, "Vstart"=-0.5, "Vstop"=0.5, "Vpoints"=10.0, "Settling"=0.01, "I limit"=0.1, "Log mapping"=FALSE, "Averaging"=0.0}, "CV properties"={"T"=0.0, "Vstart"=-0.5, "Vstop"=0.5, "Vpoints"=10.0, "Precision"=enum."Normal", "Test signal"=0.01, "Auto I range"=FALSE, "Test frequency"=100000.0, "I range"=-2.0, "V range"=10.0, "Log mapping"=FALSE, "Rel perm"=0.0, "Area"=0.0, "Equivalent circuit model"=0}, "DLTS properties"={"Tstart"=0.0, "Instant start"=FALSE, "Tstop"=0.0, "T rate"=0.0, "Test signal"=0.0, "Test frequency"=0.0, "Bandwidth"=0.0, "Averaging"=0.0, "Vbias"=0.0, "Vpulse"=0.0, "pulse length"=0.0, "Pulse 2"=FALSE, "Vpulse 2"=0.0, "pulse length 2"=0.0, "I range"=-2.0, "V range"=10.0, "Emission rate"=[], "Sampling rate"=0.0, "Acq. delay"=0.0, "Filter order"=0, "Equivalent circuit model"=0}, "LDLTS properties"={"T"=0.0, "Test signal"=0.0, "Test frequency"=0.0, "Bandwidth"=0.0, "Averaging"=0.0, "Vbias"=0.0, "Vpulse"=0.0, "pulse length"=0.0, "Pulse 2"=FALSE, "Vpulse 2"=0.0, "pulse length 2"=0.0, "I range"=-2.0, "V range"=10.0, "Sampling rate"=0.0, "Acq. delay"=0.0, "Sampling time"=0.0, "Filter order"=0, "Equivalent circuit model"=0}}}, "CV"={"Name"="", "Comment"="", "Time"=timestamp(0 s since 1904-01-01), "Folder"=path "", "CV properties"={"T"=0.0, "Vstart"=0.0, "Vstop"=0.0, "Vpoints"=0.0, "Precision"=enum."Low (Fast)", "Test signal"=0.0, "Auto I range"=FALSE, "Test frequency"=0.0, "I range"=0.0, "V range"=0.0, "Log mapping"=FALSE, "Rel perm"=0.0, "Area"=0.0, "Equivalent circuit model"=0}, "GUID"=""}}, Variant=w586) -> (data=w583:cluster{"Settings":T9, "CV":T22}, error out=w585:errorcluster)
        n208 = Unbundle By Name(w577) -> ("Settings.MFIA.Use compensation"=w575:bool, "MFIA handle.ziHandle"=w576:T19, "MFIA handle.Selected device"=w505:string)
        n209 = Unbundle By Name(w523) -> ("Binary"=w522:bool)
        n210 = Unbundle By Name(w583) -> ("CV.CV properties.Vstart"=w566:dbl[unit], "CV.CV properties.Vstop"=w563:dbl[unit], "CV.CV properties.Vpoints"=w539:dbl, "CV.CV properties.Log mapping"=w561:bool, "CV.CV properties.Precision"=w571:enum16{"Low (Fast)", "Normal", "High (Slow)"}, "CV.CV properties.Equivalent circuit model"=w493:u16, "CV.CV properties.Auto I range"=w582:bool, "CV.CV properties.Test signal"=w525:dbl[unit], "CV.CV properties.V range"=w581:dbl[unit], "CV.CV properties.I range"=w579:dbl, "CV.CV properties.Test frequency"=w531:dbl[unit])
        n211 = Cast Unit Bases(0:w525) -> (2:w524:dbl)  [unwired: 1 in]
        n212 = Cast Unit Bases(0:w581) -> (2:w580:dbl)  [unwired: 1 in]
        n213 = Power Of 10(x=w579) -> (10^x=w578:dbl)
        n214 = Bundle By Name(cluster=T29 {"model"=0, "auto/output"=FALSE, "output/amplitude"=0.1, "current/range"=0.001, "voltage/range"=1.0, "auto/inputrange"=FALSE, "mode"=1} ("Parameters"), "model"=w493, "auto/output"=FALSE, "auto/inputrange"=w582, "output/amplitude"=w524, "voltage/range"=w580, "current/range"=w578) -> (w573:T29)
        n215 = Cast Unit Bases(0:w531) -> (2:w530:dbl)  [unwired: 1 in]
        n216 = call "Set Measurment Parameters(SubVI).vi"("Handle In"=w576, "Parameters"=w573, "Pause time"=u32 300, "Error In"=w585, "Enable compensation"=w575) -> ("Handle Out"=w532:T19, "Error Out"=w535:errorcluster)
        n217 = call-poly <instrlib>:"ziSetValue.vi"("Error In"=w535, "Value"=w530, "Path"="imps/0/freq", "Handle In"=w532) -> ("Error Out"=w534:errorcluster, "Handle Out"=w533:T19)  [unwired: 1 in]
        n218 = Build Array(w505, "sigouts/0/offset" ("element")) -> (w569:string[])
        n219 = call <instrlib>:"ziModStart.vi"("Error In"=w534, "module Id"=w572, "Handle In"=w533) -> ("Error Out"=w501:errorcluster, "ModHandle Out"=w504:T20)  [unwired: 6 in, 1 out]
        n220 = call-poly <instrlib>:"ziModSetValue.vi"("Error In"=w501, "Values"=w569, "Paths"=string[] ["sweep/device", "sweep/gridnode"], "ModHandle In"=w504) -> ("Error Out"=w502:errorcluster, "ModHandle Out"=w503:T20)  [unwired: 6 in]
        n221 = Cast Unit Bases(0:w563) -> (2:w564:dbl)  [unwired: 1 in]
        n222 = Boolean To (0,1)(Boolean=w561) -> (0, 1=w562:i16)
        n223 = Cast Unit Bases(0:w566) -> (2:w565:dbl)  [unwired: 1 in]
        n224 = call "Set Precision(SubVI).vi"("Error In"=w502, "Precision"=w571, "ModHandle In"=w503) -> ("Error Out"=w500:errorcluster, "ModHandle Out"=w499:T20)  [unwired: 3 in]
        n225 = Build Array(w565, w564, w539, 0.0 ("element"), w562) -> (w567:dbl[])
        n226 = call-poly <instrlib>:"ziModSetValue.vi"("Error In"=w500, "Values"=w567, "Paths"=string[] ["sweep/start", "sweep/stop", "sweep/samplecount", "sweep/endless", "sweep/xmapping"], "ModHandle In"=w499) -> ("Error Out"=w558:errorcluster, "ModHandle Out"=w557:T20)  [unwired: 6 in]
        n227 = call <instrlib>:"ziModSubscribe.vi"("Error In"=w558, "Path"="imps/0/sample", "ModHandle In"=w557) -> ("Error Out"=w555:errorcluster, "ModHandle Out"=w554:T20)  [unwired: 6 in]
        n228 = call <instrlib>:"ziModExecuteTimeout.vi"("Error In"=w555, "Timeout 5000ms"=w507, "Modal (F)"=TRUE, "ziModHandle In"=w554) -> ("Error Out"=w552:errorcluster, "ziModHandle Out"=w551:T20)  [unwired: 4 in, 1 out]
        n229 = while {
          shift-right: [w614] -> w550
          shift-left: w552 -> [w611]
          shift-right: [w613] -> w549
          shift-left: w551 -> [w610]
          tunnel: w498 -> [w597]
          tunnel: [w589] -> w543
          tunnel: [w588] -> w494
          stop <- w595 stop-if-true
          w592 = dbl[] []
          n230 = call <instrlib>:"ziModStatus.vi"("Error In"=w611, "ModHandle IN"=w610) -> ("Error Out"=w601:errorcluster, "Finished?"=w609:bool, "Progress (unity)"=w600:dbl, "ModHandle Out"=w608:T20)  [unwired: 5 in]
          n231 = Wait on Occurrence(2:w597, 3:1000 ("ms timeout (-1)")) -> (0:w594:bool)  [unwired: 1 in]
          n232 = Not(x=w594) -> (.not. x?=w593:bool)
          n233 = Multiply(x=w600, y=100.0) -> (x*y=w599:dbl)
          n234 = Or(x=w609, y=w593) -> (x .or. y?=w595:bool)
          n235 = Format Into String(format string="Acquiring C-V profile\n(%d %%)", error in=w601, w599) -> (resulting string=w604:string, error out=w605:errorcluster)  [unwired: 1 in]
          n236 = property on="Measurement info" class="Str"(error in=w605, "Val(Sgnl)"=w604) -> (error out=w602:errorcluster)  [unwired: 1 in, 1 out]
          n237 = call <instrlib>:"ziModRead.vi"("error in"=w602, "ziModHandle In"=w608) -> ("error out"=w607:errorcluster, "ziModHandle Out"=w606:T20)  [unwired: 8 in]
          n238 = while {
            shift-right: [w619] -> w614
            shift-left: w607 -> [w631]
            shift-right: [w624] -> w613
            shift-left: w606 -> [w630]
            shift-right: [w621] -> w591
            shift-left: w592 -> [w622]
            shift-right: [w620] -> w590
            shift-left: w592 -> [w623]
            stop <- w629 stop-if-true
            n239 = call <instrlib>:"ziModGetNextNode.vi"("Error In"=w631, "ModHandle In"=w630) -> ("Error Out"=w625:errorcluster, "ModResults"=w627:T31, "ModHandle Out"=w626:T20, "NoData"=w629:bool)  [unwired: 6 in]
            n240 = Unbundle By Name(w627) -> ("ValueType"=w628:T32)
            n241 = case shown="False" w629 {
              tunnel: w628 -> [w641 _]
              tunnel: w627 -> [w640 _]
              tunnel: w626 -> [w639 w665]
              tunnel: w625 -> [w638 w664]
              tunnel: [w637 w664] -> w619
              tunnel: [w636 w665] -> w624
              tunnel: [w635 w662] -> w620
              tunnel: [w634 w663] -> w621
              tunnel: w623 -> [w633 w662]
              tunnel: w622 -> [w632 w663]
              frame False {
                n242 = case shown="\"SWEEPER_DATA\"" w641 {
                  tunnel: w640 -> [_ w657]
                  tunnel: w639 -> [w644 w656]
                  tunnel: w638 -> [w645 w658]
                  tunnel: [w645 w654] -> w637
                  tunnel: [w644 w655] -> w636
                  tunnel: [w642 w650] -> w635
                  tunnel: [w643 w649] -> w634
                  tunnel: w633 -> [w642 w648]
                  tunnel: w632 -> [w643 w647]
                  frame "NONE", Default {
                    n243 = Wait (ms)(milliseconds to wait=u32 100) -> ()  [unwired: 1 out]
                  }
                  frame "SWEEPER_DATA" {
                    n244 = call-poly <instrlib>:"ziModGetData.vi"("Error In"=w658, "ModResults"=w657, "ModHandle In"=w656) -> ("Error Out"=w654:errorcluster, "SweeperImpedanceWaveArray"=w653:T34[], "ModHandle Out"=w655:T20)  [unwired: 4 in, 2 out]
                    n245 = for {
                      tunnel: w653 -> [w661] mode=indexing
                      tunnel: [w660] -> w652 mode=concatenating
                      tunnel: [w659] -> w651 mode=concatenating
                      n246 = Unbundle By Name(w661) -> ("grid"=w659:dbl[], "param1"=w660:dbl[])
                    }
                    n247 = Build Array (concatenate)(w647, w651) -> (w649:dbl[])
                    n248 = Build Array (concatenate)(w648, w652) -> (w650:dbl[])
                  }
                }
              }
              frame True {
              }
            }
          }
          n249 = for {
            tunnel: w591 -> [w618] mode=indexing
            tunnel: w590 -> [w617] mode=indexing
            tunnel: [w618] -> w589 mode=indexing if=w615
            tunnel: [w617] -> w588 mode=indexing if=w615
            # "Filter NaNs"
            n250 = Not A Number/Path/Refnum?(number/path/refnum=w618) -> (NaN/Path/Refnum?=w616:bool)
            n251 = Not(x=w616) -> (.not. x?=w615:bool)
          }
          n252 = Bundle(w589, w588) -> (→"C-V":cluster{dbl[], dbl[]})  [unwired: 1 in]
        }
        n253 = local read "Workspace"() -> (w544:path)
        n254 = Select(t="CV.bin", s=w522, f="CV.dat") -> (s? t:f=w547:string)
        n255 = Build Path(base path=w544, name or relative path="Folder") -> (appended path=w548:path)
        n256 = Build Path(base path=w548, name or relative path=w547) -> (appended path=w540:path)
        n257 = Build Array(w543, w494) -> (w542:dbl[][])
        n258 = call <instrlib>:"ziModFinish.vi"("Error In"=w550, "ziModHandle In"=w549) -> ("Error Out"=w538:errorcluster)  [unwired: 7 in, 1 out]
        n259 = Transpose 2D Array(2D array=w542) -> (transposed array=w541:dbl[][])
        n260 = property on="Measurement info" class="Str"(error in=w538, "Val(Sgnl)"="Done!" ("Value (Signaling)")) -> (error out=w536:errorcluster)  [unwired: 1 in, 1 out]
        n261 = call "Write data file (SubVI).vi"("error in"=w536, "Binary"=w522, "2D data"=w541, "file path in"=w540) -> ("error out"=w508:errorcluster)  [unwired: 6 in, 1 out]
        n262 = property on="Export" class="Bool"(error in=w508, "Visible"=TRUE) -> (error out=w521:errorcluster)  [unwired: 1 in, 1 out]
        n263 = local read "Rel perm"() -> (w515:dbl)
        n264 = property on="Measure" class="Bool"(error in=w521, "BoolText.Text"="Remeasure" ("Boolean Text.Text"), "DisabledEnum"=w518) -> (error out=w519:errorcluster)  [unwired: 1 in, 1 out]
        n265 = local read "Area"() -> (w517:dbl[unit])
        n266 = Cast Unit Bases(0:w517) -> (2:w516:dbl)  [unwired: 1 in]
        n267 = Cast Unit Bases(0:w515) -> (2:w514:dbl)  [unwired: 1 in]
        n268 = property on="Calculate" class="Bool"(error in=w519, "DisabledEnum"=w518) -> (error out=w497:errorcluster)  [unwired: 1 in, 1 out]
        n269 = Not Equal To 0?(x=w516) -> (x != 0?=w513:bool)
        n270 = Not Equal To 0?(x=w514) -> (x != 0?=w512:bool)
        n271 = And(x=w513, y=w512) -> (x .and. y?=w511:bool)
        n272 = property on="Stop" class="Bool"(error in=w497, "DisabledEnum"=T24."Disabled and Grayed Out" ("Disabled")) -> (error out=w496:errorcluster)  [unwired: 1 in, 1 out]
        n273 = case shown="True" w511 {
          tunnel: w496 -> [w666 w670]
          tunnel: [w666 w669] -> w510
          tunnel: w509 -> [_ w668]
          frame False {
          }
          frame True {
            n274 = Generate User Event(user event=w668, event data cluster=TRUE ("event data"), error in=w670) -> (error out=w669:errorcluster)  [unwired: 1 in, 1 out]
          }
        }
      }
      frame "Stop" {
        n275 = Generate User Event(user event=w674, event data cluster=TRUE ("event data"), error in=w675) -> (error out=w672:errorcluster)  [unwired: 1 in, 1 out]
      }
    }
    n276 = call <vilib>:"General Error Handler.vi"("type of dialog (OK msg:1)"=w480, "error in (no error)"=w482) -> ("error out"=w481:errorcluster)  [unwired: 9 in, 4 out]
    n277 = call <vilib>:"Clear Errors.vi"("error in (no error)"=w481) -> ("error out"=w478:errorcluster)  [unwired: 5 in, 1 out]
  }
  n278 = Unregister For Events(event registration refnum=w49, error in=w50) -> (error out=w20:errorcluster)
  n279 = Destroy User Event(user event=w18, error in=w20) -> (error out=w19:errorcluster)
  n280 = Destroy User Event(user event=w46, error in=w19) -> (error out=w31:errorcluster)
  n281 = Merge Errors(w31, w29) -> (w30:errorcluster)
  n282 = Release Queue(queue=w47, error in (no error)=w30) -> (error out=→"Error Out":errorcluster)  [unwired: 1 in, 2 out]
